vi "HEWH File Setup.vi"(0 "Data File Directory":path=path "D:/Data", 1 "Test_Type:":string(combo)="Stand Override", 2 "Station":string, 5 "error in (no error)":errorcluster, 7 "File Extension:":string="csv") -> (15 "FileInit Cluster":T8={"Scan Rate Adjust"=1000.0, "Draw Count"=0, "Test Patten Setup"={"Dispense Times"=[0.0, 3600.0, 7200.0, 10800.0, 14400.0, 18000.0], "Total Gallons Schedule"=[10.72, 10.72, 10.72, 10.72, 10.72, 10.72], "Flow Rate Schedule "=[3.0, 3.0, 3.0, 3.0, 3.0, 3.0], "Incoming Water Temperature"=[58.0, 58.0, 58.0, 58.0, 58.0, 58.0], "PreDraw Pattern"=[], "24 Hour PreDraw"=enum."Zero Pre-Draws", "Pre-Draw Until?"=[], "Purge Until Cutout"=FALSE, "Heating Flag"=FALSE}, "Condition Cluster Output"={"Condition #1"=FALSE, "Condition #2"=FALSE, "Special Last Draw (HU Test)"=FALSE, "RTD Out Temperature <="=0.0, "Condition #3"=FALSE, "Mean Tank Temperature <="=0.0, "Condition #4"=FALSE, "Decrease Outlet Temperature \nBy (RTD Out)"=0.0, "Condition #5"=FALSE, "Condition #6"=FALSE, "Time (Seconds)"=0.0, "Condition #7"=FALSE, "Condition #8"=FALSE, "Draw Until Condition"={"UE"=FALSE, "LE"=FALSE, "COMP"=FALSE, "FANS"=FALSE}, "Condition #9"=FALSE}, "HEWH Specific DAQ"={"HEWH Data"={"Voltage (Volts)"=-1.0, "Current (Amps)"=-1.0, "Power (Watts)"=-1.0, "WattHours (Wh)"=-1.0, "TC Tree (AVG)"=0.0, "Flow Rate (GPM)"=0.0, "Gallons (Gal)"=0.0, "RTD Out (Deg F)"=0.0, "TC Down"=0.0, "TC Tree Array"=[], "UE Event Lead"=0, "LE Event Lead"=0}, "Intellif Valve % Open"=0.0, "Power State"={"UE"=FALSE, "LE"=FALSE, "COMP"=FALSE, "FANS"=FALSE}, "Power Analyzer"=enum."APLUS", "Intellifaucet Configuration"=enum."DRK375,STATION3,1/2\"HOSE"}, "Test Output Data"={"PreDraw Data Table"=[], "Data Table"=[], "MW100 TC Headers"=[]}, "Calc and Calibration"={"RTD Max Min Array"=[], "Draw Statistics"=[], "Calibration Coefficients DBL"=[], "Min RTD Temp\nDuring Draw"=0.0, "Start Gallons"=0.0, "Starting Temp Decline Temp"=0.0, "Max RTD Temp\nDuring Draw"=0.0, "Draw Start Time"=0.0, "Delay Start Time"=0.0, "Current Purge Start Time"=0.0}, "Current Draw Time"=0.0} {"Test Patten Setup"."Incoming Water Temperature" format="%.2f"; "Test Patten Setup"."Flow Rate Schedule" format="%.2f"; "Test Patten Setup"."Total Gallons Schedule" format="%.2f"; "Test Patten Setup"."Dispense Times" format="%<%H:%M:%S>t"}, 19 "error out":errorcluster)   [LabVIEW 2016]
uses:
  Hybrid Water Heater/Type Definitions/HEWH Output Information.ctl
  Hybrid Water Heater/Type Definitions/HEWH Power Data.ctl
  Hybrid Water Heater/Type Definitions/HEWH Draw Pattern Setup.ctl
  Hybrid Water Heater/Type Definitions/HEWH Power Elements.ctl
  Hybrid Water Heater/Type Definitions/HEWH Termination Condition Cluster.ctl
  GEA2 Commands/HEWH/Type Definitions/GEA2 Commands.ctl
  Type Definitions/UTILITY Power Analyzer.ctl
  Hybrid Water Heater/Custom Instrument Control/Intellifaucet/Type Definitions/INTELLIFAUCET Tested Flowrate Scenarios.ctl
  File Setup.lvlib
  Type Definition/Save File DOE LabView Program.ctl
  LabVIEW GEA2 Toolkit v1.0.0.0/library/GEA2_Toolkit.lvlib
  Hybrid Water Heater/Type Definitions/HEWH Start Conditions.ctl
  Hybrid Water Heater/Support VIs/Draw Water Specific/Type Definitions/Terminate Draw Conditions.ctl
  Type Definition/Save File HEWH Heating Control Mode.ctl
  Hybrid Water Heater/Type Definitions/PRAT Test.ctl
  Hybrid Water Heater/Support VIs/Draw Water Specific/Type Definitions/HEWH Special Condition Check.ctl
  Hybrid Water Heater/Support VIs/Draw Water Specific/Type Definitions/Check Special Condtions.ctl
  Hybrid Water Heater/Type Definitions/HEWH Draw Flag ENUM.ctl
  Custom Pallet Controls/Custom Pallet String.ctl
  Custom Pallet Controls/Custom Pallet Forward.ctl
  Hybrid Water Heater/Type Definitions/HEWH PreDraw.ctl
  <vilib>/Platform/fileVersionInfo.llb/FileVersionInformation.ctl
  Type Definition/Save File DISH Dishwasher Details.ctl
  Type Definition/DPT IMC Data.ctl
  Washer DOE/Type Definitions/DOE Appliance Common.ctl
  Washer DOE/Type Definitions/DOE Dryer Standard.ctl
panel:
  in  "Appliance Details":T1={"FileVersionInfo"={"FileVersion"="", "ProductName"="", "InternalName"="", "CompanyName"="", "LegalCopyright"="", "FileDescription"=""}, "Dishwasher Info"={"Open Cup Weight (gm):"=0.0, "Auto Cup Weight (gm):"=0.0, "Detergent-Dish:"="", "Inlet Temperature-Dish:"="", "Cycle Mode-Dish:"="", "Unit Control-Dish:"="", "Manufacturer-Dish:"=""}, "Washer Info"={"Hot Water Temperature (Fahrenheit):"="", "Cold Water Temperature (Fahrenheit):"="", "Capacity (cu.ft):"=0.0, "Initial Cloth Weight:"=0.0, "Cloth Lot:"=0, "Model Family:"="", "Program Name:"="", "Cycle Selection:"="", "Wash Temperature:"="", "Rinse Temperature:"="", "Load Size:"=""}, "File Name Output Array"=[], "Calibration Output Array"=[], "Appliance Common"={"Engineer:"="", "Model Number:"="", "Serial Number:"="", "Comments:"="", "Station ID:"="", "Technician:"="", "TR Number:"="", "Lab ID:"="", "Voltage:"="", "Water Pressure (PSI):"="", "Test Date:"="", "Computer Name:"="", "IP Address:"="", "Ambient RH:"="", "Frequency:"="", "Build:"="", "Filename:"="", "Test Type:"="", "Load Run #:"=0, "Ambient Temperature (F):"="", "File Path:"=path "", "Cycles Per Year"=60}, "Water Heater"={"Heating Mode:"=""}, "Dryer"={"Heat Setting:"="", "Washer Water Temperature (60 ± 5°F):"=60, "Water Hardness (PPM):"=17, "Dryness Setting:"="", "Dryer Type:"="", "Exhaust:"="", "Drying Cycle:"="", "Load Type:"="", "Nominal Load Weight"="", "Dryer Initial IMC Data"={"Measured IMC (lbs)"=7.0, "Actual Initial RMC (%)"=7.0, "RMC (Desired %)"=100.0, "Bone Dry Wt(lbs)"=7.0, "Tolerance(%)"=5.0, "Actual Final RMC (%)"=7.0, "CEF (lbf/kWh)"=0.0, "Minimum Weight (lbf)"=0.0, "Average Weight (lbf)"=0.0, "Maximum Weight (lbf)"=0.0, "Measured IMC In Range?"=FALSE, "Moisture Reduction Factor"=55.5, "Field Use Factor"=1.04, "Empty Dryer Cold Weigth"=0.0, "Energy Standard"=enum."D2-Automatic Dryer", "Weight Cloth (lbs)"=0.0, "Relative Moisture Content (%)"=0.0, "Relative Moisture Content - Avg (%)"=0.0}}} {"Dryer"."Dryer Initial IMC Data"."Maximum Weight (lbf)" format="%03_6g"; "Dryer"."Dryer Initial IMC Data"."Average Weight (lbf)" format="%03_6g"; "Dryer"."Dryer Initial IMC Data"."Minimum Weight (lbf)" format="%03_6g"; "Dryer"."Dryer Initial IMC Data"."CEF (lbf/kWh)" format="%03_6g"; "Dryer"."Dryer Initial IMC Data"."Actual Final RMC (%)" format="%03_6g"; "Dryer"."Dryer Initial IMC Data"."Tolerance(%)" format="%0#_6g"; "Dryer"."Dryer Initial IMC Data"."Bone Dry Wt(lbs)" format="%03_6g"; "Dryer"."Dryer Initial IMC Data"."RMC (Desired %)" format="%0#_6g"; "Dryer"."Dryer Initial IMC Data"."Actual Initial RMC (%)" format="%03_6g"; "Dryer"."Dryer Initial IMC Data"."Measured IMC (lbs)" format="%0#_6g"}
  in  "Technician:":string(combo)
  in  "Lab ID:":string(combo)
  in  "TR Number:":string(combo)
  in  "Get Serial Number":bool
  in  "Get Model Number":bool
  in  "Supply Voltage":string(combo)
  in  "Heating Mode:":string(combo)
  out "Description":string="File Name Setup"
  in  "Model:":T4
  in  "Ambient Temp SetPoint:":string(combo)
  in  "Engineer:":T4
  in  "Comments:":string
  in  "Test Name:":T4
  in  "OK":T7
  in  "Serial Number:":T4
  in  "Ambient RH:":string(combo)
  in  "Build:":string(combo)
  in  "Frequency:":string(combo)
  in  "Test Station":T4
  in  "Tab Control":enum32{"Location Data", "Output Data"}(tab)
  out "Unhandled Error":errorcluster
  out "FileName":path
  out "Filename":string
  out "OutputData":string[][](array[string])
  # "Select Only One Condition"
  # "Just Draw Water!"
  # "Condition #1"
  # "Draw Until Any Heat Source"
  # "Condition #2"
  # "Start Dispense Pattern"
  # "Draw Until Specific Heat Source"
  # "Condition #3"
  # "Dispense PRAT Sequence"
  # "Not Working"
  # "Condition #4"
  # "Condition #5"
  # "Condition #6"
  # "Draw Pattern Setup"
  # "Pre-Draw Items"
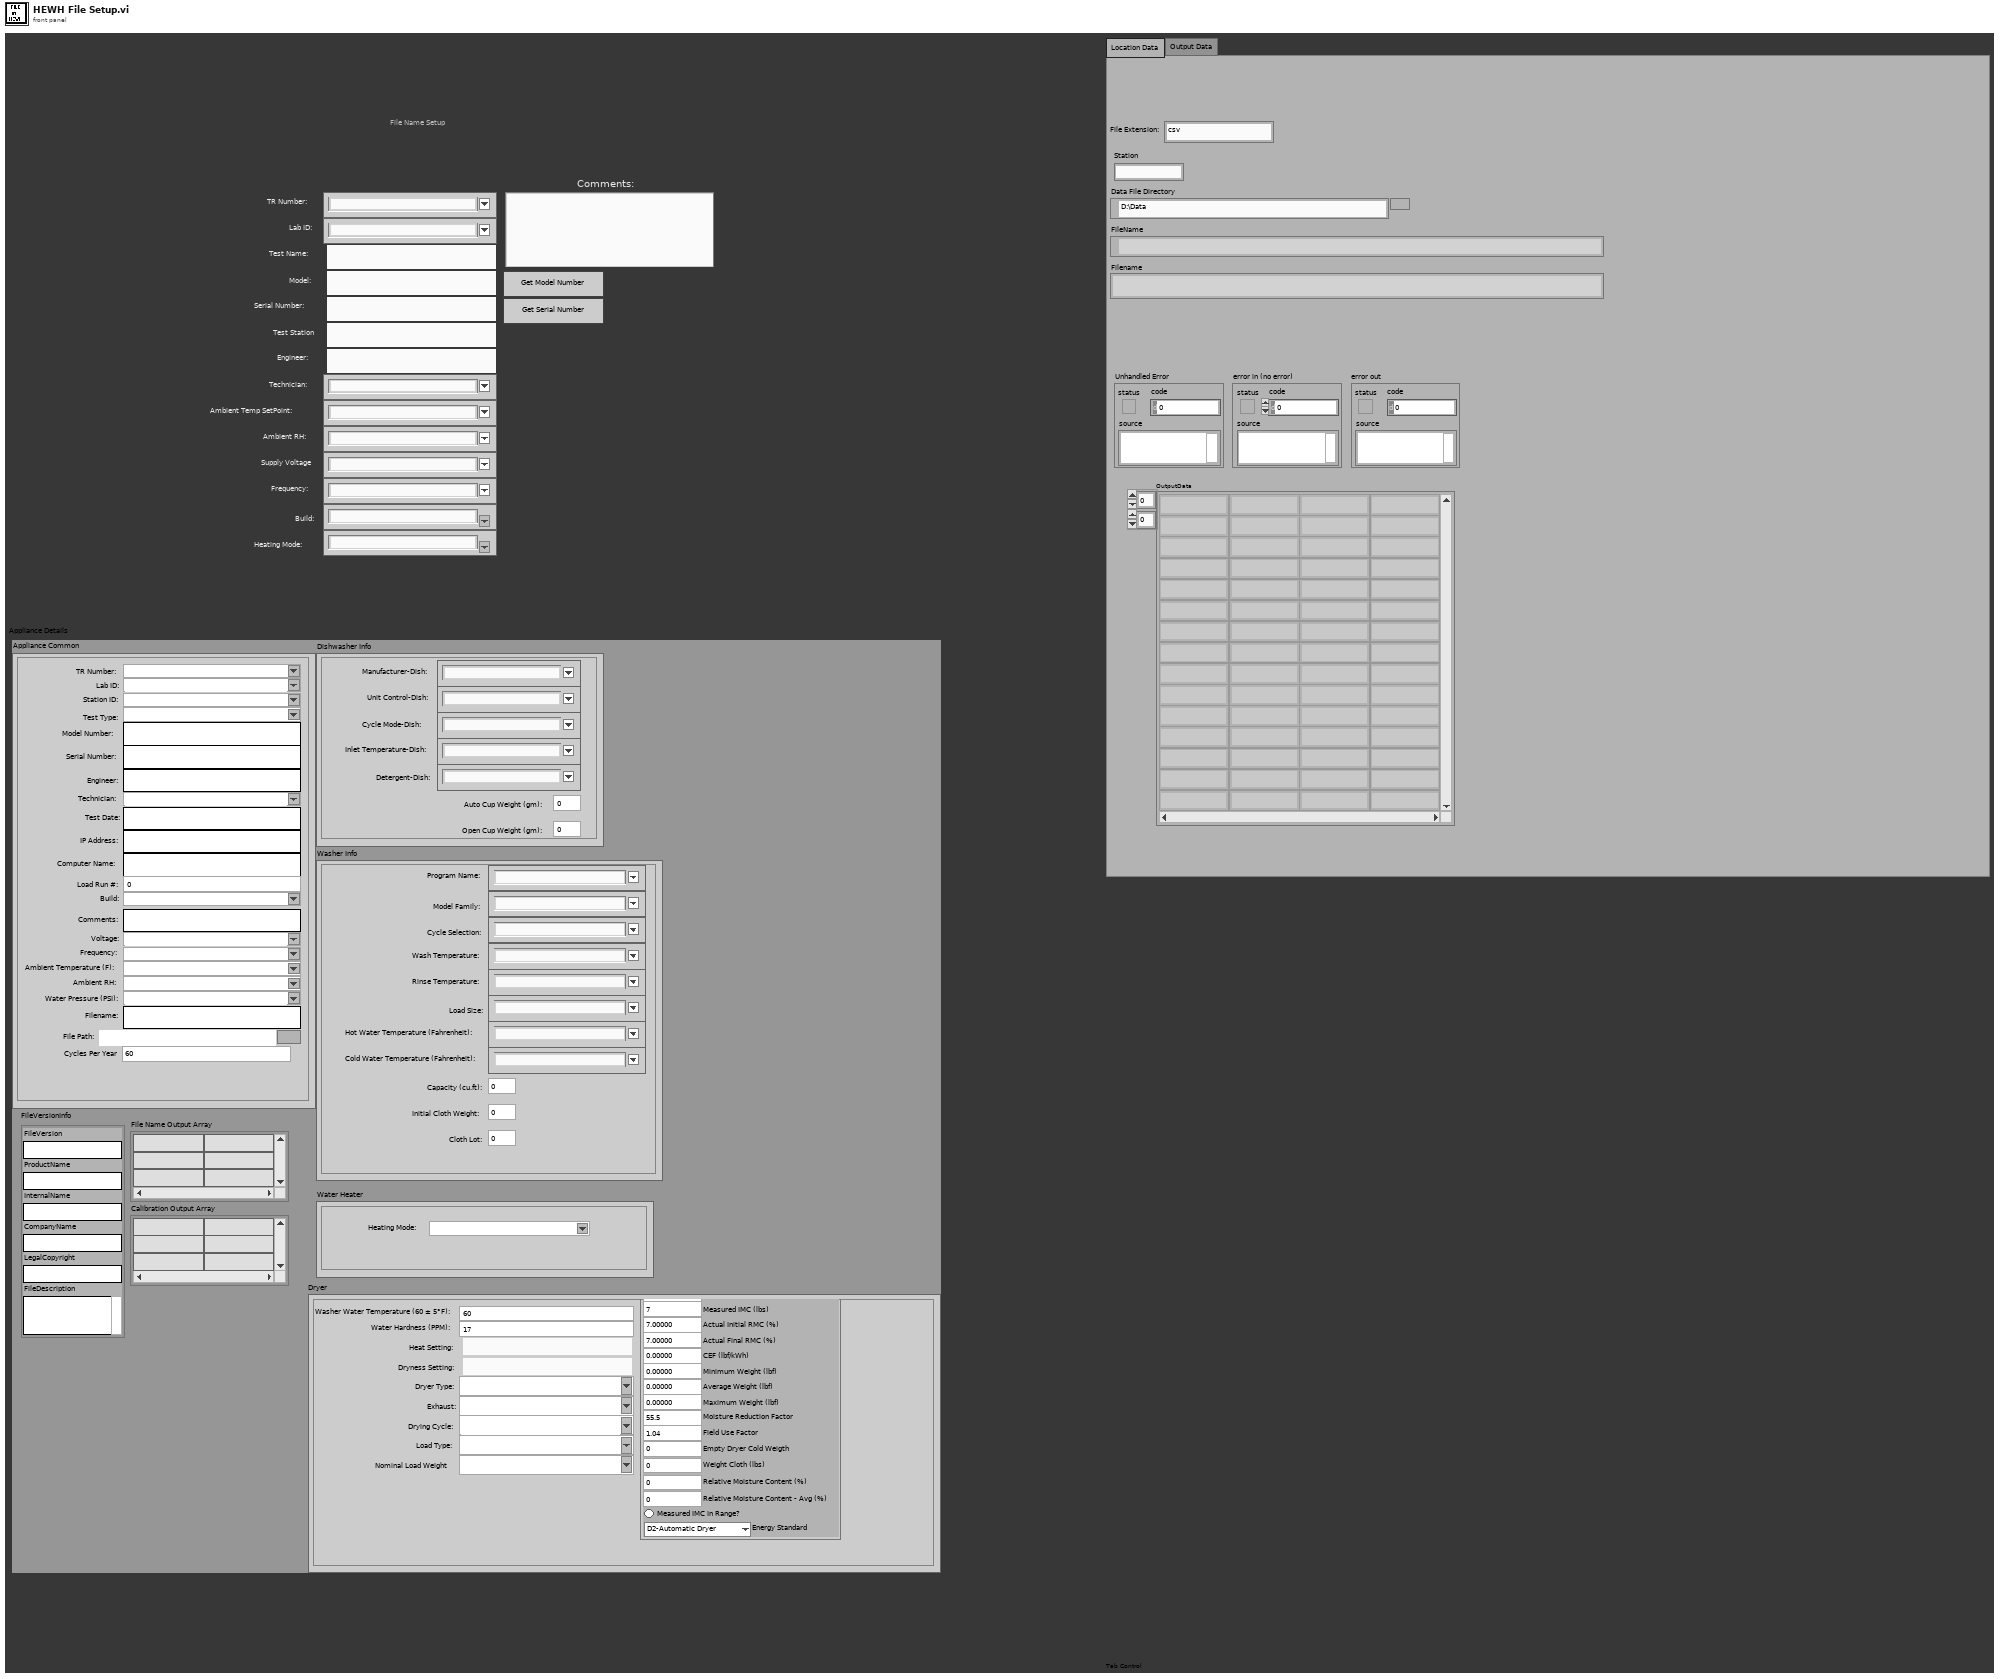
[diagram p1: front panel]
types:
  T1 = typedef "File Setup.lvlib/Save File DISH Dishwasher Details.ctl" = cluster{"FileVersionInfo":T2, "Dishwasher Info":cluster{"Open Cup Weight (gm):":dbl, "Auto Cup Weight (gm):":dbl, "Detergent-Dish:":string, "Inlet Temperature-Dish:":string, "Cycle Mode-Dish:":string, "Unit Control-Dish:":string, "Manufacturer-Dish:":string}, "Washer Info":cluster{"Hot Water Temperature (Fahrenheit):":string, "Cold Water Temperature (Fahrenheit):":string, "Capacity (cu.ft):":dbl, "Initial Cloth Weight:":dbl, "Cloth Lot:":i32, "Model Family:":string, "Program Name:":string, "Cycle Selection:":string, "Wash Temperature:":string, "Rinse Temperature:":string, "Load Size:":string}, "File Name Output Array":string[][], "Calibration Output Array":string[][], "Appliance Common":T3, "Water Heater":cluster{"Heating Mode:":string}, "Dryer":cluster{"Heat Setting:":T4, "Washer Water Temperature (60 ± 5°F):":u16, "Water Hardness (PPM):":u16, "Dryness Setting:":T4, "Dryer Type:":string, "Exhaust:":string, "Drying Cycle:":string, "Load Type:":string, "Nominal Load Weight":string, "Dryer Initial IMC Data":T5}}
  T2 = typedef "FileVersionInformation.ctl" = cluster{"FileVersion":string, "ProductName":string, "InternalName":string, "CompanyName":string, "LegalCopyright":string, "FileDescription":string}
  T3 = typedef "DOE Appliance Common.ctl" = cluster{"Engineer:":string, "Model Number:":string, "Serial Number:":string, "Comments:":string, "Station ID:":string, "Technician:":string, "TR Number:":string, "Lab ID:":string, "Voltage:":string, "Water Pressure (PSI):":string, "Test Date:":string, "Computer Name:":string, "IP Address:":string, "Ambient RH:":string, "Frequency:":string, "Build:":string, "Filename:":string, "Test Type:":string, "Load Run #:":i32, "Ambient Temperature (F):":string, "File Path:":path, "Cycles Per Year":u32}
  T4 = typedef "Custom Pallet String.ctl" = string
  T5 = typedef "DPT IMC Data.ctl" = cluster{"Measured IMC (lbs)":dbl, "Actual Initial RMC (%)":dbl, "RMC (Desired %)":dbl, "Bone Dry Wt(lbs)":dbl, "Tolerance(%)":dbl, "Actual Final RMC (%)":dbl, "CEF (lbf/kWh)":dbl, "Minimum Weight (lbf)":dbl, "Average Weight (lbf)":dbl, "Maximum Weight (lbf)":dbl, "Measured IMC In Range?":bool, "Moisture Reduction Factor":dbl, "Field Use Factor":dbl, "Empty Dryer Cold Weigth":dbl, "Energy Standard":T6, "Weight Cloth (lbs)":dbl, "Relative Moisture Content (%)":dbl, "Relative Moisture Content - Avg (%)":dbl}
  T6 = typedef "DOE Dryer Standard.ctl" = enum16{"D2-Automatic Dryer", "D2-Timer Dryer", "D1-Automatic Dryer", "D1-Timer Dryer", "Other"}
  T7 = typedef "Custom Pallet Forward.ctl" = bool
  T8 = typedef "HEWH Output Information.ctl" = cluster{"Scan Rate Adjust":dbl, "Draw Count":i32, "Test Patten Setup":T9, "Condition Cluster Output":T11, "HEWH Specific DAQ":cluster{"HEWH Data":T13, "Intellif Valve % Open":dbl, "Power State":T12, "Power Analyzer":T14, "Intellifaucet Configuration":T15}, "Test Output Data":cluster{"PreDraw Data Table":string[][], "Data Table":string[][], "MW100 TC Headers":string[]}, "Calc and Calibration":cluster{"RTD Max Min Array":dbl[][], "Draw Statistics":dbl[][], "Calibration Coefficients DBL":dbl[][], "Min RTD Temp\nDuring Draw":dbl, "Start Gallons":dbl, "Starting Temp Decline Temp":dbl, "Max RTD Temp\nDuring Draw":dbl, "Draw Start Time":dbl, "Delay Start Time":dbl, "Current Purge Start Time":dbl}, "Current Draw Time":dbl}
  T9 = typedef "HEWH Draw Pattern Setup.ctl" = cluster{"Dispense Times":dbl[], "Total Gallons Schedule":dbl[], "Flow Rate Schedule ":dbl[], "Incoming Water Temperature":dbl[], "PreDraw Pattern":dbl[][], "24 Hour PreDraw":T10, "Pre-Draw Until?":bool[], "Purge Until Cutout":bool, "Heating Flag":bool}
  T10 = typedef "HEWH PreDraw.ctl" = enum16{"Zero Pre-Draws", "One Pre- Draws", "Two Pre-Draws", "Three Pre-Draws", ""}
  T11 = typedef "HEWH Termination Condition Cluster.ctl" = cluster{"Condition #1":bool, "Condition #2":bool, "Special Last Draw (HU Test)":bool, "RTD Out Temperature <=":dbl, "Condition #3":bool, "Mean Tank Temperature <=":dbl, "Condition #4":bool, "Decrease Outlet Temperature \nBy (RTD Out)":dbl, "Condition #5":bool, "Condition #6":bool, "Time (Seconds)":dbl, "Condition #7":bool, "Condition #8":bool, "Draw Until Condition":T12, "Condition #9":bool}
  T12 = typedef "HEWH Power Elements.ctl" = cluster{"UE":bool, "LE":bool, "COMP":bool, "FANS":bool}
  T13 = typedef "HEWH Power Data.ctl" = cluster{"Voltage (Volts)":dbl, "Current (Amps)":dbl, "Power (Watts)":dbl, "WattHours (Wh)":dbl, "TC Tree (AVG)":dbl, "Flow Rate (GPM)":dbl, "Gallons (Gal)":dbl, "RTD Out (Deg F)":dbl, "TC Down":dbl, "TC Tree Array":dbl[], "UE Event Lead":i32, "LE Event Lead":i32}
  T14 = typedef "UTILITY Power Analyzer.ctl" = enum16{"", "APLUS", "WT210", "WT500", "WT300", "OSI", "Debug", "WT230", "WT300_1", "WT300_2"}
  T15 = typedef "INTELLIFAUCET Tested Flowrate Scenarios.ctl" = enum16{"DRK500,Station1", "DRK375,Lab", "SRK500,Station1,5GPM FR", "DRK375,STATION3,1/2\"HOSE", "DRK500,Station1,downspout", "DRK375,Station3,thruEcocute", "DRK375,Station3,purge", "Build2,2B,Purge", "Global, Purge", "Global, Tank", "DRK250"}
  T16 = enum32{"invalid app kind", "Development System", "Run Time System", "Student Edition", "Embedded LabVIEW", "Evaluation", "Custom"}
  T17 = enum32{"Invalid", "Standard", "Closed", "Hidden", "Minimized", "Maximized"}
  T18 = typedef "File Setup.lvlib/Save File DOE LabView Program.ctl" = enum16{"No Name Found", "DOE Stand", "Dishwasher Kitchen", "Portable Stand", "HEWH", "Dryer", "Dryer WILT", "HCC", "PRAT", "HEWH RLT"}
  T19 = typedef "GEA2 Commands.ctl" = enum16{"CMD_CANCEL_EEV_POSITION", "CMD_CLEAR_ENERGY_USAGE_CTRS", "CMD_CLEAR_FAULT_COUNTS", "CMD_CLEAR_OVERRIDE_STATUS", "CMD_COMP_OFF", "CMD_COMP_ON", "CMD_DSM_OVERRIDES", "CMD_EEV_POSITION", "CMD_ENTER_EXIT_FCT_MODE", "CMD_ENTER_FACT_MODE", "CMD_HP_RUN_6MIN", "CMD_INITIATE_REMOTE_DSM_OVERRIDE", "CMD_LE_2_SECONDS", "CMD_REFRESH_SERVICE_TIMEOUTS", "CMD_RESET", "CMD_RESET_FILTER_TIMES", "CMD_RESTORE_EEPROM_DEFAULTS", "CMD_RQST_LED_STATUS", "CMD_SET_AMBIENT_THRESH_1", "CMD_SET_AMBIENT_THRESH_2", "CMD_SET_AMBIENT_THRESH_3", "CMD_SET_CURRENTS", "CMD_SET_EEV_DRIVE_LINES", "CMD_SET_EEV_STOP_POSITION", "CMD_SET_LEDS", "CMD_SET_MODEL_NUMBER", "CMD_SET_PID_I_DENOM_OVER_THR", "CMD_SET_PID_I_DENOM_UNDER_THR", "CMD_SET_PID_LOW_SH_TARGET", "CMD_SET_PID_MID_SH_TARGET", "CMD_SET_PID_P_DENOMINATOR", "CMD_SET_SERIAL_NUMBER", "CMD_SET_START_POS_OVER_THR", "CMD_SET_START_POS_UNDER_THR", "CMD_TOGGLE_FAN", "CMD_TOGGLE_LE_SERV", "CMD_TOGGLE_SERVICE_MODE", "CMD_TOGGLE_UE_SERV", "CMD_TURN_ON_OFF_DLB", "CMD_UE_2_SECONDS", "CMD_UPDATE_DSM_LEVEL", "CMD_UPDATE_MODE", "CMD_WRITE_SETPOINTS", "REQ_READ_KEY_STATUS", "REQ_SYSTEM_MODE", "RQST_CURRENT_PID_SH_TARGET", "RQST_DATA_FROM_DATA_FLASH", "RQST_DATA_FROM_MEMORY", "RQST_DSM_OVERRIDE_STATUS", "RQST_HEM_KWH_DATA", "RQST_HYPERTERM_OUTPUT_DATA", "RQST_IDLB_RESISTANCE", "RQST_MODEL_NUMBER", "RQST_MODEL_SELECT_AD_VALUE", "RQST_OTHER_FAULT_COUNTS", "RQST_OVERRIDE_STATUS", "RQST_PID_PARAMETERS", "RQST_READ_PERSONALITY", "RQST_SERIAL_NUMBER", "RQST_SERVICE_ERROR_CODES", "RQST_Software_Version", "RQST_SS_FAULT_COUNTS", "RQST_STATUS_QUERY", "RQST_STD_ELEC_RANGE", "RQST_SUPPORTED_MODES", "RQST_T2_RESISTANCE", "RQST_T3B_RESISTANCE", "RQST_T4_RESISTANCE", "RQST_T5_RESISTANCE", "RQST_TEMP_RANGE", "RQST_VACATION_RANGE", "RQST_WATER_CAPACITY"}
  T20 = typedef "GEA2_Toolkit.lvlib/Data In.ctl" = cluster{"Source":u8, "Destination":u8, "Command":u8, "Message":string}
  T21 = typedef "GEA2_Toolkit.lvlib/Data Out.ctl" = cluster{"Source":u8, "Destination":u8, "Command":u8, "Length":u8, "CRC":u16, "Message":string}
  T22 = typedef "ViperHawk Data.ctl" = cluster{"GEA Diagnostic Data - Washer":T23, "Software Version":T24, "Debug Search Parameters":T25, "Message Count":i32, "Number of Messages":i32, "Partial Message String":string, "Full Message to Save":string, "Board ID":string, "Board Index":i32, "Source Address":u8, "Destination Address":u8, "Data to send":u8[], "ReceivedData":u8[], "Debug/GEA Data":string[], "Command":u8, "GEA2 Reference Out":refnum<k24>, "GEA2 Event Registration":refnum<event-registration>, "Bus Data":string, "GEA Data":string[][], "Network Variable Location":i32, "Water Heater GEA2 Data":T26}
  T23 = typedef "ViperHawk Diagnostic Data.ctl" = cluster{"Speed (RPM)":u32, "Load Size":u32, "Temperature":u32, "Water Pressure":dbl, "Detergent":u32, "Fabric Softener":u32, "Tub Direction":string, "Detergent Valve":bool, "Fabric Softener Valve":bool, "Recirculating Pump":bool, "Drain Valve":bool, "Hot Valve":bool, "Cold Valve":bool, "Lid Closed Status":string, "Lid Lock Status":string, "Error Count":u32, "IGBT Temperature (Deg C)":u32, "Motor Speed":u32, "Latched OOB":u32, "Raw OOB":u32, "Plaster Status":u32, "Inverter Power (W)":u32, "Target Speed(BRPM)":u32, "Latched Agitate Motor Temp (Deg C)":u32, "Current Motor Temp (Deg C)":u32, "Profiler Status":string, "Current Inverter Action":string, "Error Codes":string, "Lid Locked":bool, "Lid Closed":bool, "9E Diagnostic Data":cluster{"Total Cycle Time (Min)":u32, "Total Cycle Count (Current)":u16, "Total Error Count":u16, "Machine Error History":u32, "Washer UI History":u32, "Inverter Error History":u32, "Cycle Storage Limit":u8, "Error Storage Limit":u8, "Cycle Pages Supported":u8, "Error Pages Supported":u8, "Inverter Reset Count":u16}, "9F Diagnostic Data":cluster{"Cycle Buffer Index":string, "Page Number":string, "Total Cycle Count":u32, "Delay Start Time":u32, "Stain Selected":string, "Selected Cycle":u32, "eWash":string, "Soil Level":string, "Temperature":string, "Overnight Ready":string, "Spin Setting":string, "Control Lock Status":string, "Stain Remover":string, "Steam Assist":string, "My Cycle":string, "PreWash":string, "Debug Log Enabled":string, "Rinse":string, "Signal Level":string, "PreSoak":string}}
  T24 = typedef "Save File.lvlib/Save File Software Version.ctl" = cluster{"Critical Major SW Version":string, "Critical Minor SW Version":string, "Major SW Version":string, "Minor SW Version":string, "Parametric Data Ver. Major":string, "Parametric Data Ver. Minor":string, "Diagnostics Data Ver. Major":string, "Diagnostics Data Ver. Minor":string, "Current Personality Setting":string}
  T25 = typedef "ViperHawk Search Control.ctl" = cluster{"Pause":string[], "Run":string[], "EOC":string[], "Error Codes":string[]}
  T26 = typedef "GEA2 Commands WaterHeater GEA2 Data.ctl" = cluster{"GEA2 Label Array":string[], "PID_PARAMETERS":string[][], "SUPPORTED_MODES":string[][], "Button Status":T27, "Status Query":T28, "Service Error Codes":T29, "HEM_KWH_DATA":string[][], "OTHER_FAULT_COUNTS":string[][], "GEA2 Raw Message":string, "Hyperterminal Data":cluster{"Source":u8, "Destination":u8, "Command":u8, "Length":u8, "CRC":u16, "UE - state (1/0 on off)":u8, "LE - state (1/0 on off)":u8, "Comp - state (1/0 on off)":u8, "Fan  - state (1/0 on off)":u8, "Setpoint Deg F":i32, "T2(TankSensor)":dbl, "T3A(EvapIn)":dbl, "T3B(EvapOut)":dbl, "T4(CompressorDischarge)":dbl, "T5(Ambient)":dbl, "Current":dbl, "Voltage (Volts)":u16, "EEV Position (0-480)":u16, "Reason for last heating cycle termination":u16, "Reason Data word 1":string, "Reason Data word 2":string, "Reason Data word 3":string, "Reason Data word 4":string, "SW Debug Data":string, "Flow Events (Bit Encoded)":u16, "Heating Control Mode":u16}, "Extra Data":cluster{"Water Capacity (Gallons)":u32, "Max Vacation Duration Days":u32, "Min Vacation Duration Days":u32, "Max Set Point (Deg F)":u32, "Min Set Point (Deg F)":u32, "T5 Resistance":u32, "T4 Resistance":u32, "T3B Resistance":u32, "T2 Resistance":u32, "STD_ELEC_RANGE":string, "SS_FAULT_COUNTS":string, "SERIAL_NUMBER":string, "READ_PERSONALITY":u8, "RQST_OVERRIDE_STATUS":string, "MODEL_SELECT_AD_VALUE":u32, "MODEL NUMBER":string, "IDLB_RESISTANCE":u32, "DSM Override Status":string, "RQST_DATA_FROM_Memory":string, "RQST_DATA_FROM_DATA_FLASH":string, "RQST_CURRENT_PID_SH_TARGET":u16, "Unit System Mode":string}}
  T27 = typedef "GEA2 Commands Button Status.ctl" = cluster{"Switch 1":bool, "Switch 2":bool, "Switch 3":bool, "Switch 4":bool, "Switch 5":bool, "Switch 6":bool, "Switch 7":bool, "Switch 8":bool, "Switch 9":bool, "Switch 10":bool, "Switch 11":bool, "Switch 12":bool, "Switch 13":bool, "Switch 14":bool, "Switch 15":bool, "Switch 16":bool}
  T28 = typedef "GEA2 Commands Status Query.ctl" = cluster{"Days Remaining (For Std Electric and Vacation)":u8, "Unit Status":string, "Current Tank Temp in Deg F":u8, "Current Setpoint in Deg F":u8, "Filter Status (% used)":u8, "Fallback Status (Fallback heating mode)":string, "Fallback Temp":u8, "\"Set Mode\" Selection":string}
  T29 = typedef "GEA2 Commands Service Error Codes.ctl" = cluster{"Reserved":bool, "Reserved 1":bool, "Reserved 2":bool, "Reserved 3":bool, "Reserved 4":bool, "Reserved 5":bool, "Reserved 6":bool, "Reserved 7":bool, "DataFlash Fail Status":bool, "Stuck Key Fail Status":bool, "Dry Tank Fail Status":bool, "Miswire Fail Status":bool, "Reserved 8":bool, "Reserved 9":bool, "Reserved 10":bool, "Reserved 11":bool, "UE Fail Status":bool, "LE Fail Status":bool, "Filter Fail Status":bool, "T3A Fail Status":bool, "T3B Fail Status":bool, "T4 Fail Status":bool, "T5 Fail Status":bool, "T2 Fail Status":bool, "SS Cond A Status":bool, "SS Cond B Status":bool, "SS Cond C Status":bool, "SS Cond D Status":bool, "SS Cond E Status":bool, "SS Cond F Status":bool, "SS Fan Status":bool, "CMP Fail Status":bool}
  T30 = typedef "HEWH Output Information.ctl" = cluster{"Scan Rate Adjust":dbl, "Draw Count":i32, "Test Patten Setup":T31, "Condition Cluster Output":T11, "HEWH Specific DAQ":cluster{"HEWH Data":T39, "Intellif Valve % Open":dbl, "Power State":T12, "Power Analyzer":T14, "Intellifaucet Configuration":T15}, "Test Output Data":cluster{"PreDraw Data Table":string[][], "Data Table":string[][], "MW100 TC Headers":string[]}, "Calc and Calibration":cluster{"RTD Max Min Array":dbl[][], "Draw Statistics":dbl[][], "Calibration Coefficients DBL":dbl[][], "Min RTD Temp\nDuring Draw":dbl, "Start Gallons":dbl, "Starting Temp Decline Temp":dbl, "Max RTD Temp\nDuring Draw":dbl, "Draw Start Time":dbl, "Delay Start Time":dbl, "Current Purge Start Time":dbl}, "Current Draw Time":dbl}
  T31 = typedef "HEWH Draw Pattern Setup.ctl" = cluster{"Total Gallons Schedule":dbl[], "PRAT/RLT Sequence":T32[], "Current Sequence Index":i32}
  T32 = typedef "PRAT Test.ctl" = cluster{"Sequence #":dbl, "Cycles":i32, "Mode Setting":T33, "Flow Rate (GPM)":dbl, "Temperature (F)":dbl, "Reset Timer":bool, "Use Temp Decline Method":bool, "Terminate Condition":T34, "Condition Value #1":dbl, "UE":bool, "LE":bool, "Comp":bool, "Fan":bool, "Test End Time (Sec)":dbl, "Purge Until Cutout":bool, "Start Conditions":T35, "Condition Value #2":dbl, "Remove Power":bool, "Time":dbl, "Check Special Cond.":T36, "Condition#":T37, "Draw Flags":T38, "Data Processing Delay (FHD 15sec, UEF 5 Sec)":dbl, "Test Complete":bool}
  T33 = typedef "File Setup.lvlib/Save File HEWH Heating Control Mode.ctl" = string
  T34 = typedef "Terminate Draw Conditions.ctl" = enum16{"C1-Terminate Draw @ Gallon Mark", "C2-Special Last Draw (HU Test)", "C3-RTD Out <=", "C4-Mean Tank Temp <=", "C5-Decrease RTD Out (Deg F)", "C6-Time (Seconds)", "C7-Until Any Heat Source", "C8-Specific Heat Source", "C9-Do Nothing"}
  T35 = typedef "HEWH Start Conditions.ctl" = enum16{"Heat Source Cutout", "At Time (Seconds)", "Every X (Seconds)", "T2 >= X° Below Setpoint", "Seconds From Complete", "Wait for LE & Comp Cutout", "Wait for Comp Cutout", "Wait for LE Cutout", "Wait for UE Cutout"}
  T36 = typedef "Check Special Condtions.ctl" = enum16{"SC1-Do Nothing", "SC2-Check Heat Source (On-C2/Off-C1)", "SC3-Check Skip Condition", "SC4-Check Heat Source ON/Fail"}
  T37 = typedef "HEWH Special Condition Check.ctl" = enum16{"N/A", "C1", "C2", "Reset/Fail", "Skip Draw Sequence"}
  T38 = typedef "HEWH Draw Flag ENUM.ctl" = enum16{"N/A", "None(0)", "Sml(1)", "Med(2)", "SmlMed(3)", "Lrg(4)", "SmlLrg(5)", "MedLrg(6)", "SmlMedLrg(7)"}
  T39 = typedef "HEWH Power Data.ctl" = cluster{"HEWH Standard":cluster{"Voltage (Volts)":dbl, "Current (Amps)":dbl, "Power (Watts)":dbl, "WattHours (Wh)":dbl, "TC Tree (AVG)":dbl, "Flow Rate (GPM)":dbl, "Gallons (Gal)":dbl, "RTD Out (Deg F)":dbl, "RTD In (Deg F)":dbl, "RTD Amb (Deg F)":dbl, "TC Down":dbl, "UE Event Lead":i32, "LE Event Lead":i32, "TC Tree Array":dbl[]}, "PRAT":cluster{"Power (Watts) A":dbl, "Power (Watts) B":dbl, "Power (Watts) C":dbl, "Power (Watts) D":dbl, "TC1":dbl, "TC2":dbl, "TC3":dbl, "TC4":dbl, "WattHours (Wh) A":dbl, "WattHours (Wh) B":dbl, "WattHours (Wh) C":dbl, "WattHours (Wh) D":dbl, "Ambient":dbl, "Extra Temp":dbl}, "Additional Power Data":cluster{"Vthd":dbl, "Frequency (Hz)":dbl, "Apparent Power (VA)":dbl, "Power Factor":dbl, "Current Crest Factor":dbl, "Voltage Crest Factor":dbl, "Integration Time (sec)":dbl}}
  T40 = cluster{"Core":cluster{"Current VI Reference":refnum<vi>, "Close Panel on Exit?":bool}, "Error Flag":bool, "Weights":cluster{"Measured IMC":dbl, "Actual RMC":dbl, "RMC (Desired)":dbl, "Bone Dry Wt(lbs)":dbl, "Tolerance(%)":dbl}, "HEWH Output Information":T30, "Test_Type:":string, "Supply Voltage":string, "Appliance Details":T1}
  T41 = cluster{"Measured IMC":dbl, "Actual RMC":dbl, "RMC (Desired)":dbl, "Bone Dry Wt(lbs)":dbl, "Tolerance(%)":dbl}
  T42 = cluster{"Current VI Reference":refnum<vi>, "Close Panel on Exit?":bool}
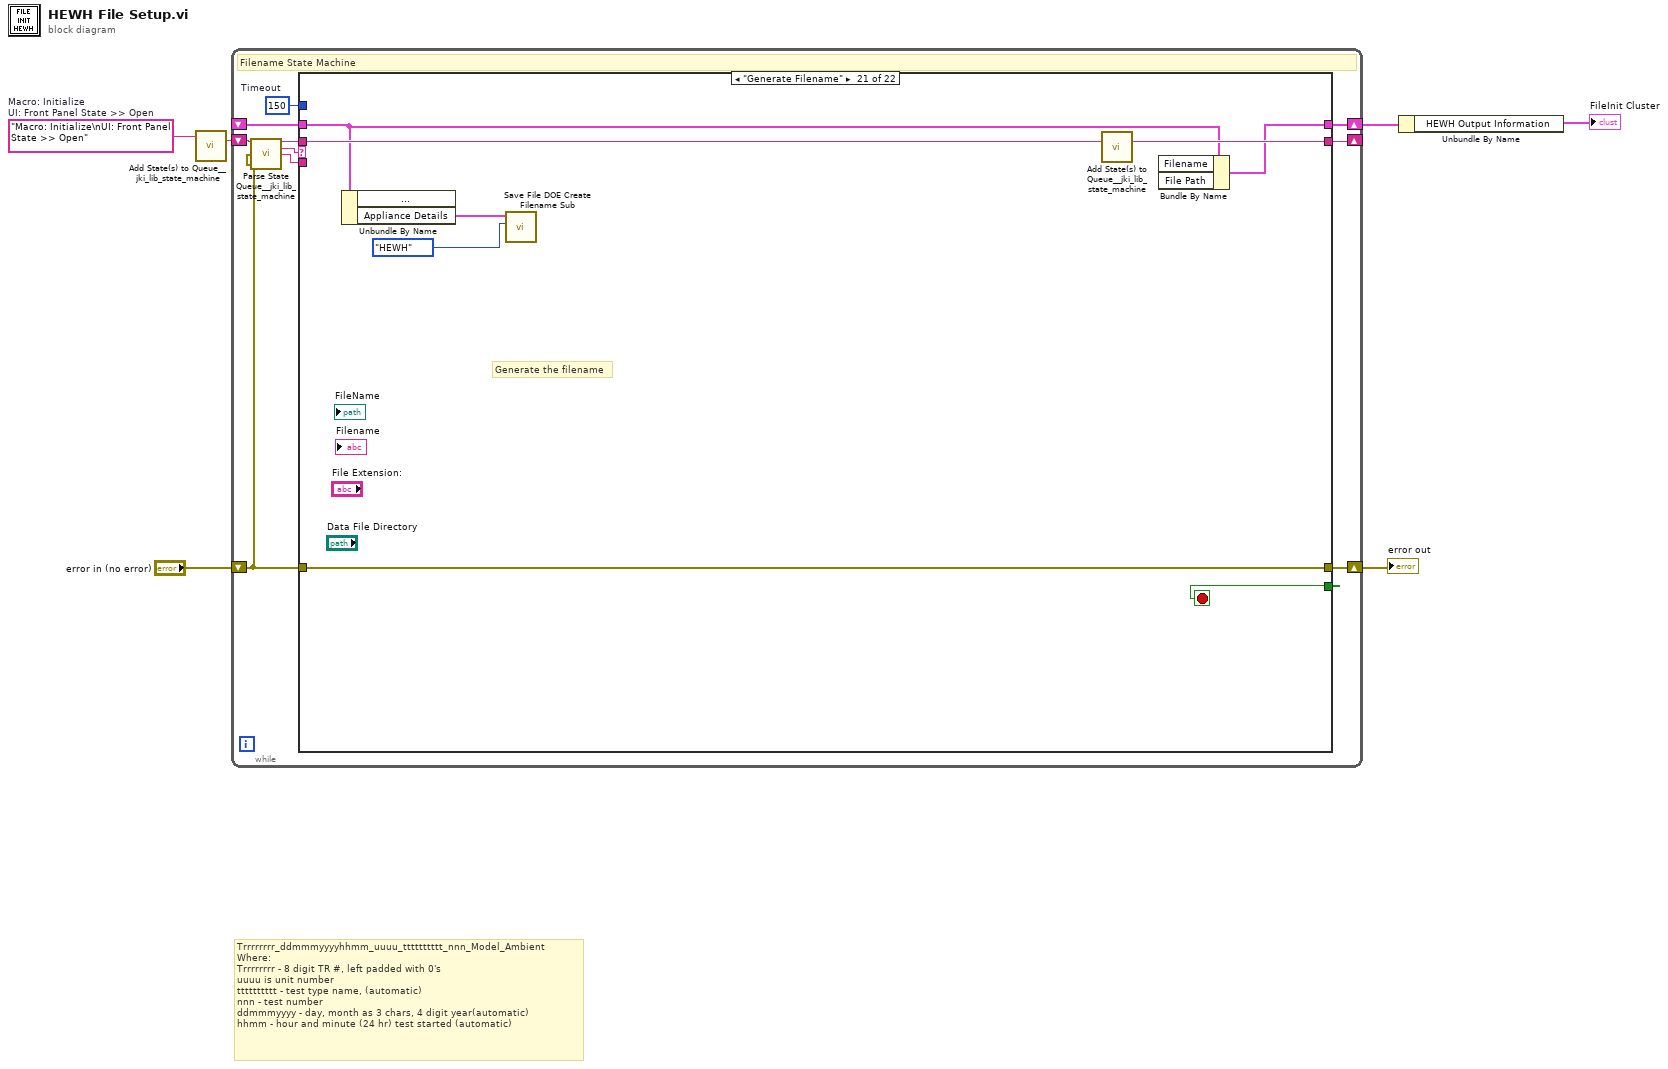
[diagram p0: block diagram]
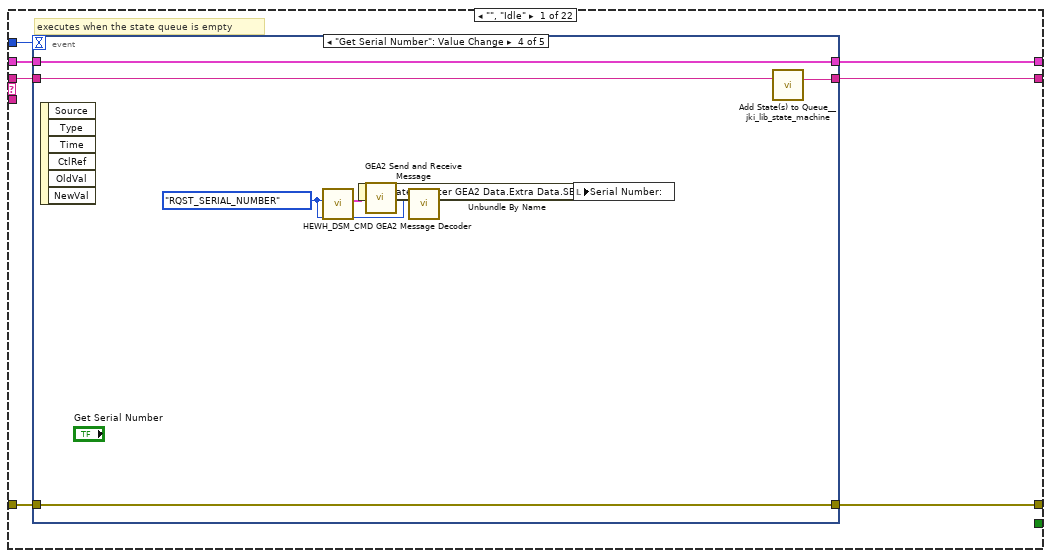
[diagram p2: hidden frame]
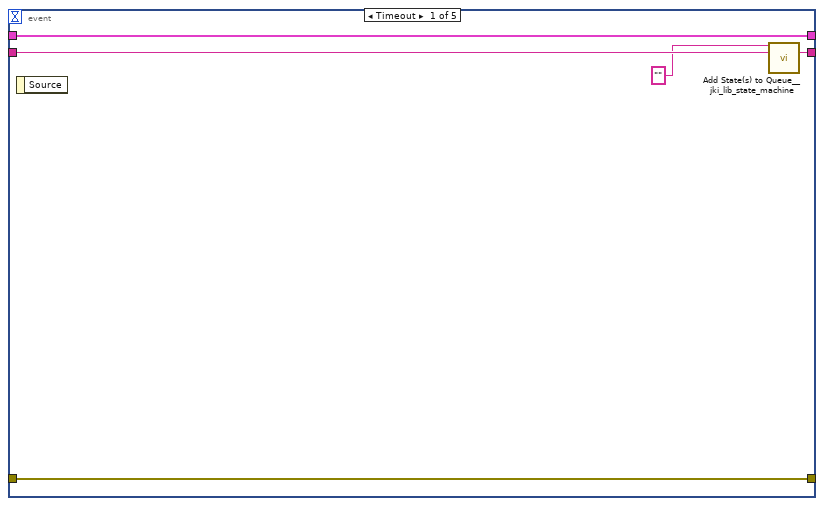
[diagram p3: hidden frame]
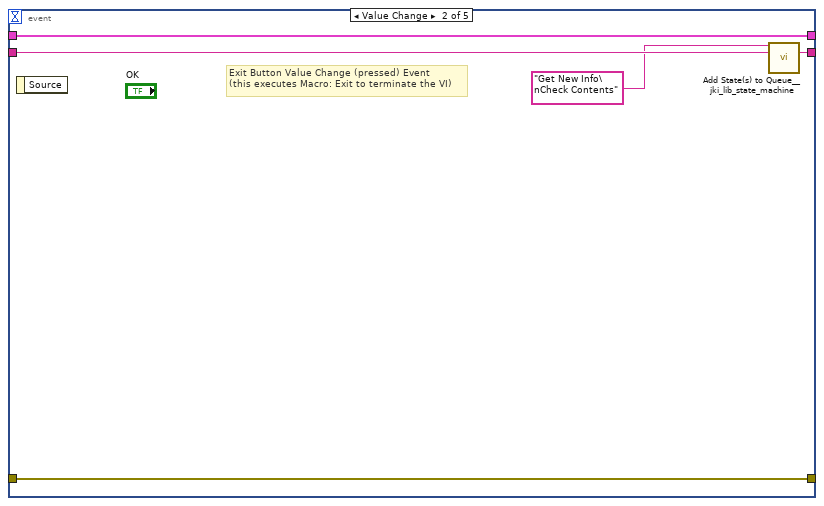
[diagram p4: hidden frame]
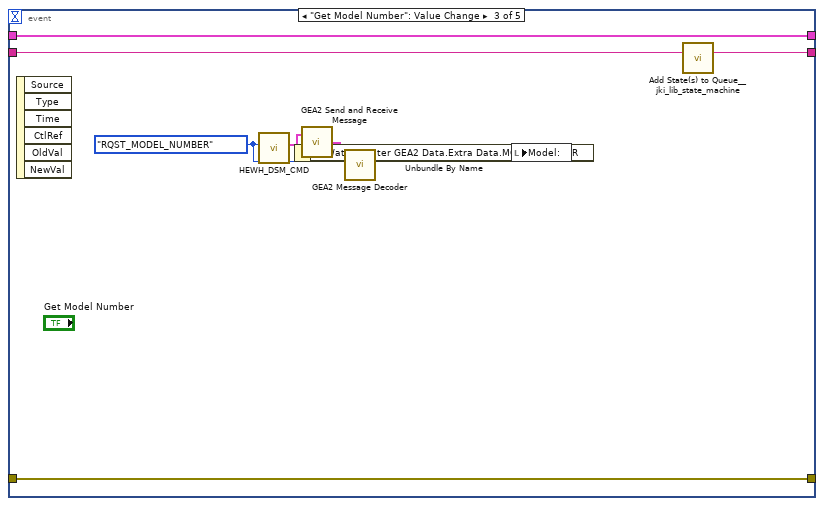
[diagram p5: hidden frame]
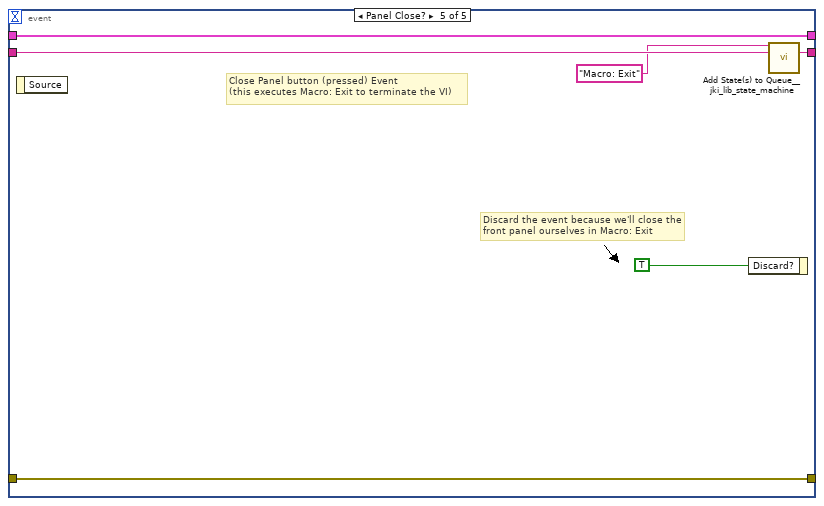
[diagram p6: hidden frame]
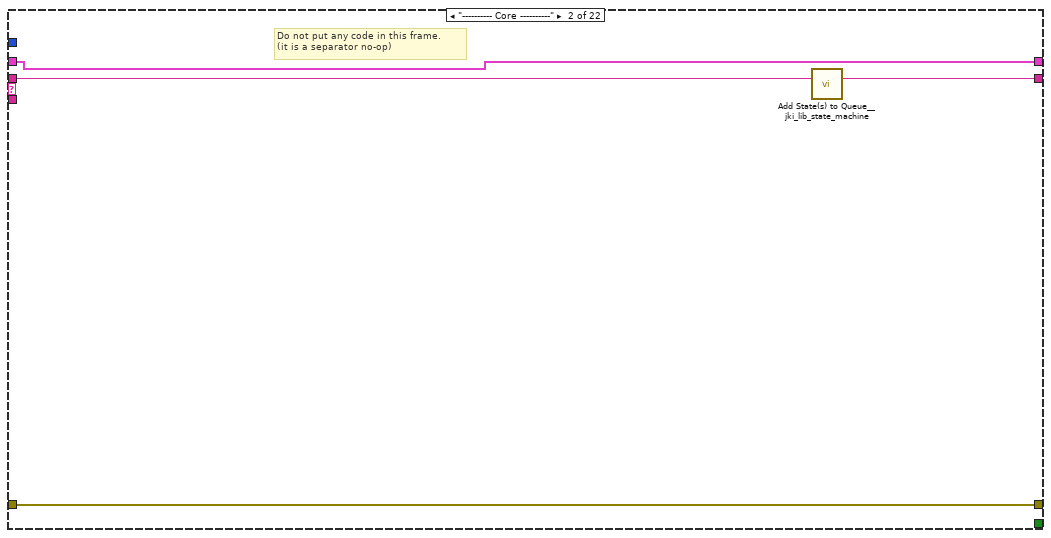
[diagram p7: hidden frame]
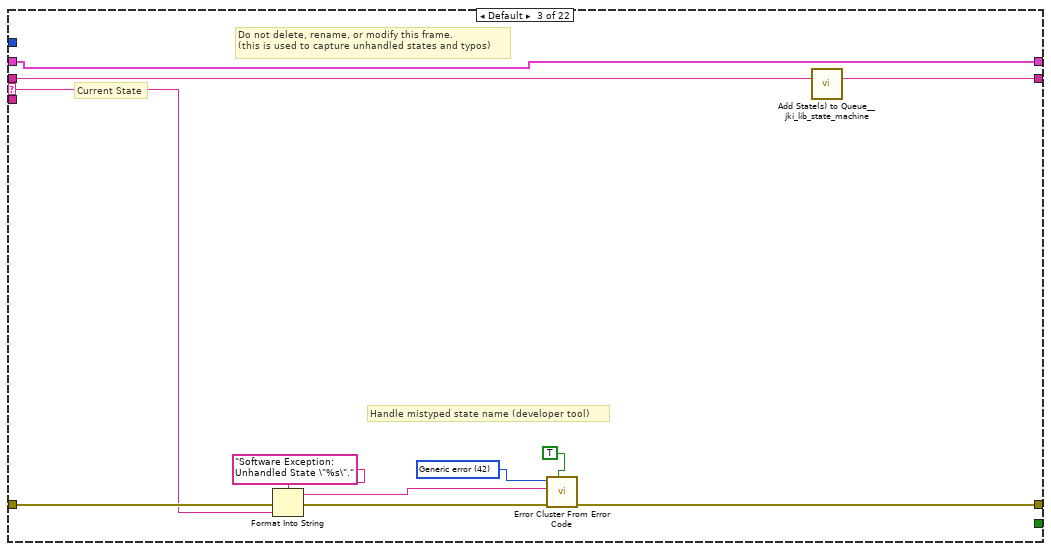
[diagram p8: hidden frame]
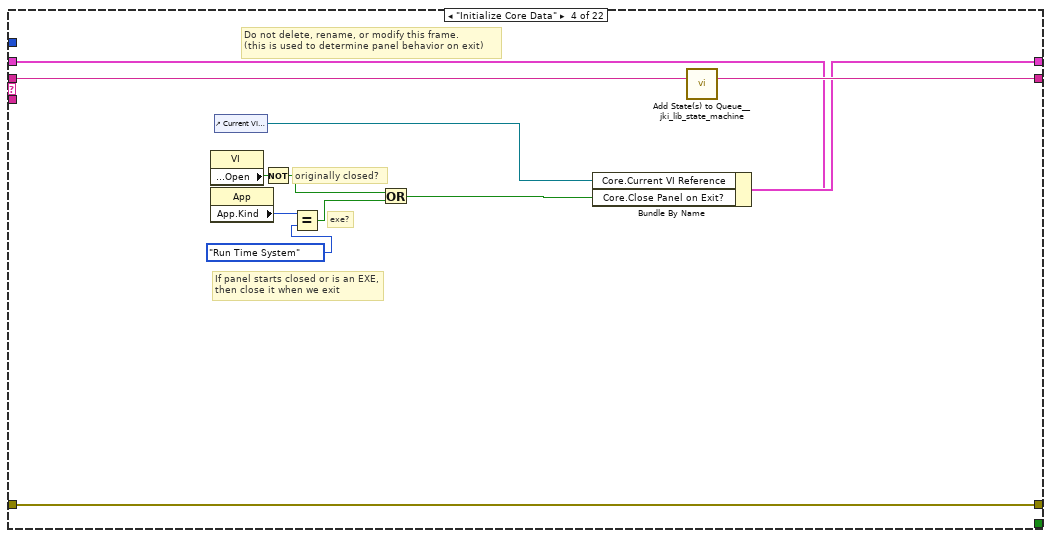
[diagram p9: hidden frame]
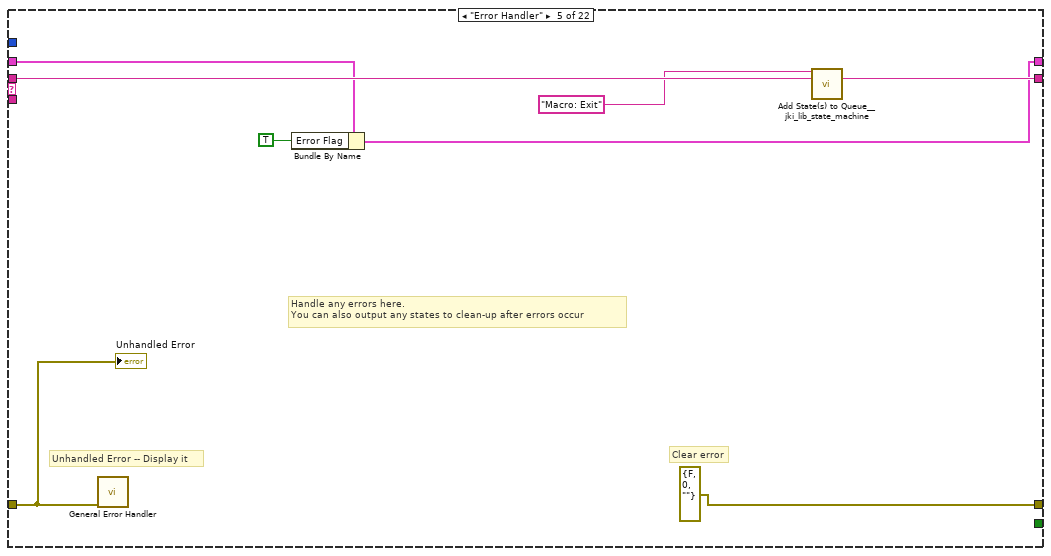
[diagram p10: hidden frame]
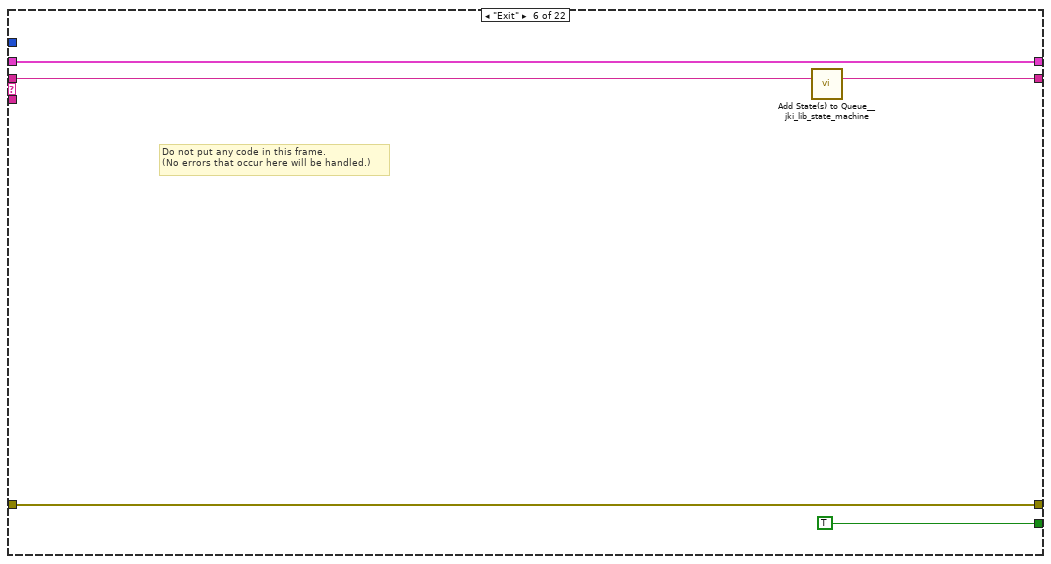
[diagram p11: hidden frame]
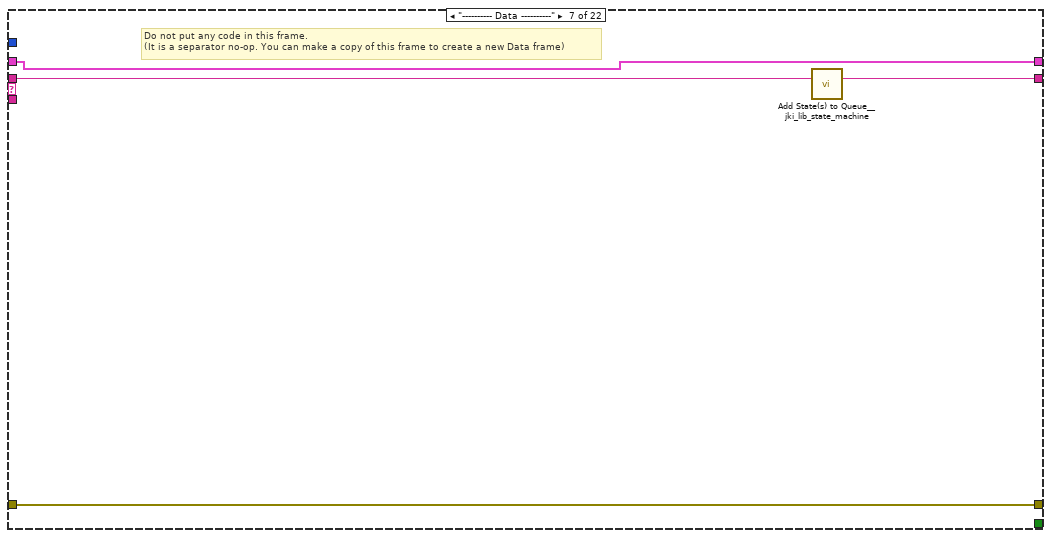
[diagram p12: hidden frame]
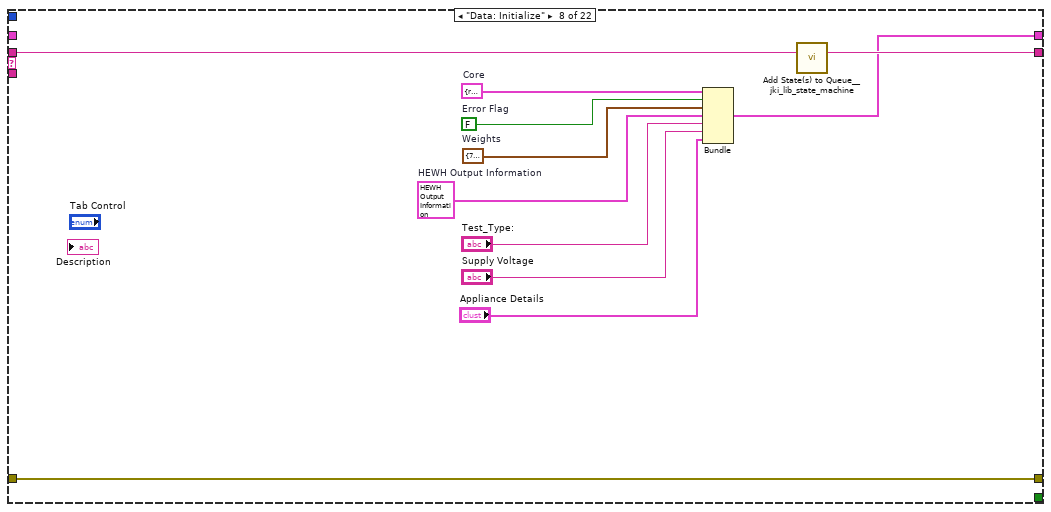
[diagram p13: hidden frame]
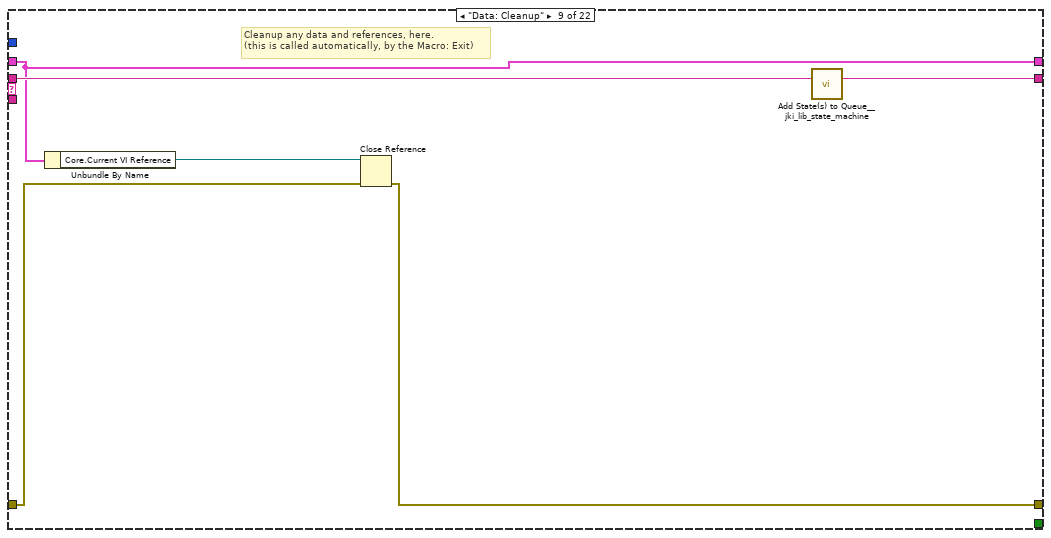
[diagram p14: hidden frame]
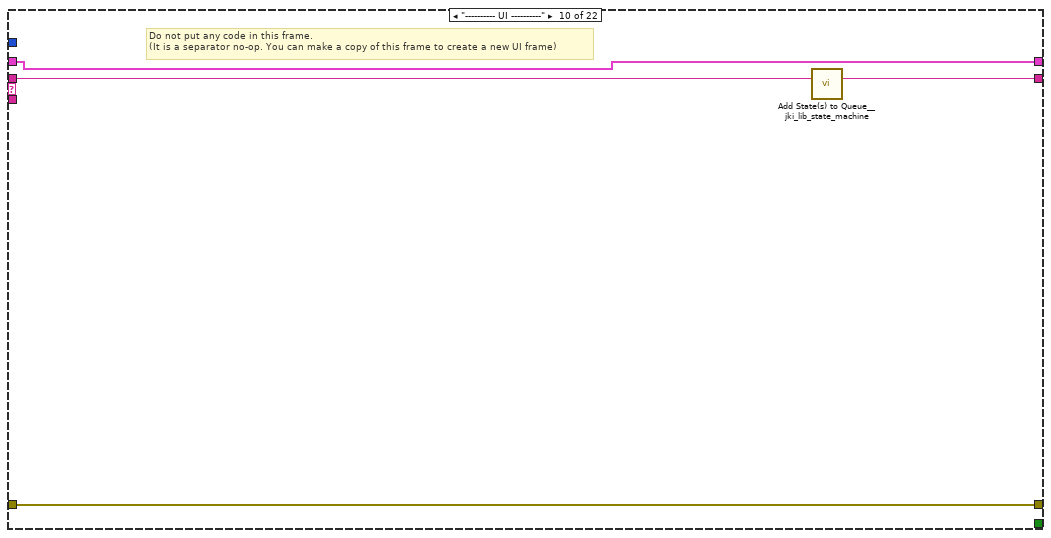
[diagram p15: hidden frame]
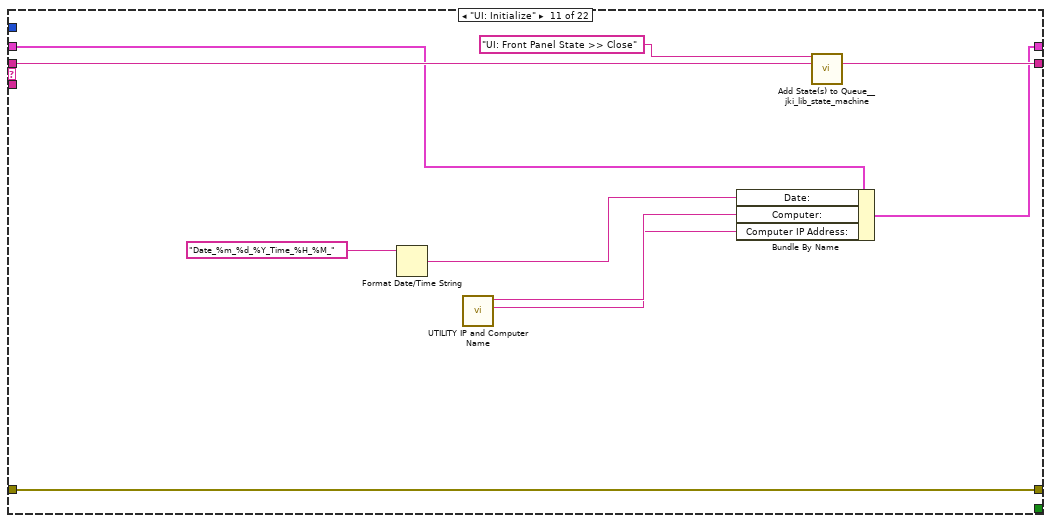
[diagram p16: hidden frame]
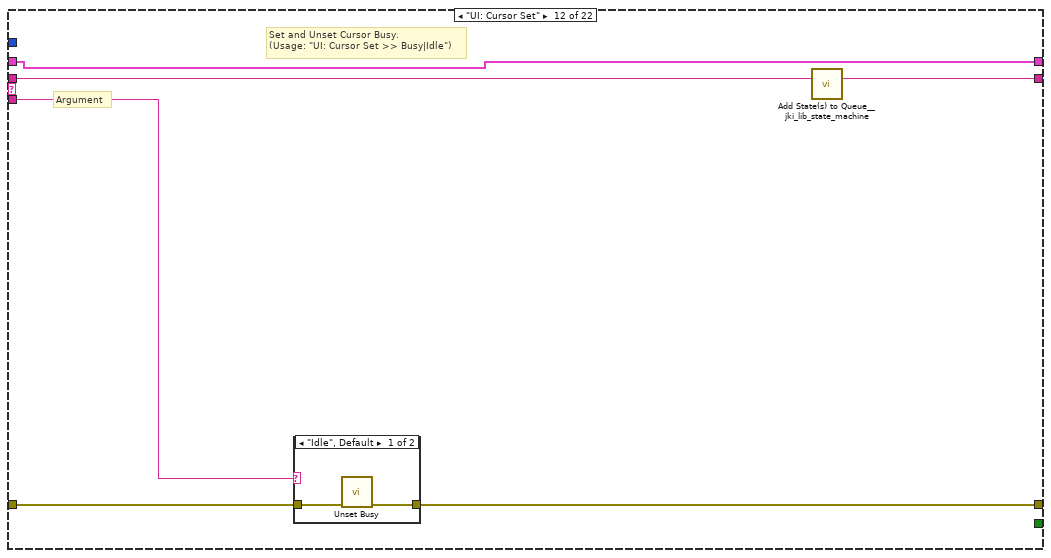
[diagram p17: hidden frame]
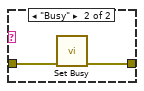
[diagram p18: hidden frame]
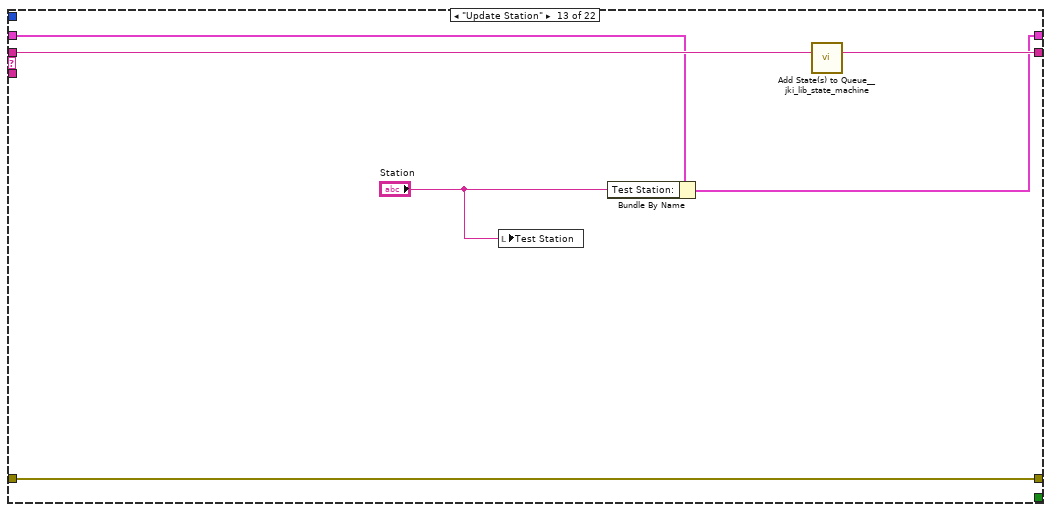
[diagram p19: hidden frame]
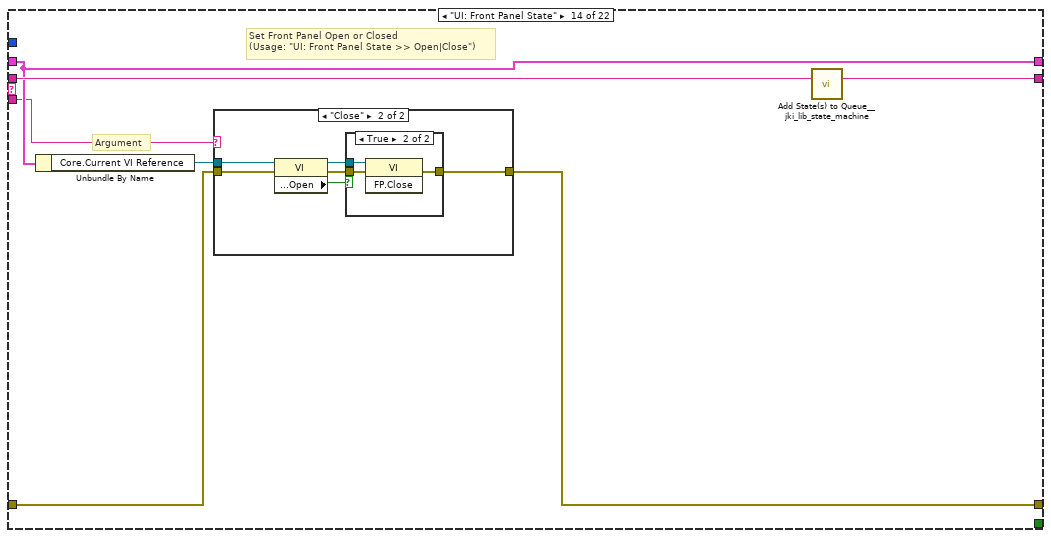
[diagram p20: hidden frame]
diagram:
  w4 = "Macro: Initialize\nUI: Front Panel State >> Open"  # Macro: Initialize UI: Front Panel State >> Open
  # "Trrrrrrrr_ddmmmyyyyhhmm_uuuu_tttttttttt_nnn_Model_Ambient\nWhere:\nTrrrrrrrr - 8 digit TR #, left padded with 0's\nuuuu is unit number\ntttttttttt - test type name, (automatic)\nnnn - test number\nddmmmyyyy - day, month as 3 chars, 4 digit year(automatic)\nhhmm - hour and minute (24 hr) test started (automatic)"
  n1 = call <vilib>:"Add State(s) to Queue__jki_lib_state_machine.vi"("State(s) in (\"\")"=w4) -> ("States Out"=w5:string)  [unwired: 14 in]
  n2 = while {
    shift-right: [w10] -> w1
    shift-left: _ -> [w9]
    shift-right: [w13] -> w6
    shift-left: "error in (no error)" -> [w7]
    shift-right: [w12] -> _
    shift-left: w5 -> [w14]
    stop <- w11 stop-if-true
    w8 = 150  # Timeout
    # "Filename State Machine"
    n3 = call <vilib>:"Parse State Queue__jki_lib_state_machine.vi"("State Queue"=w14, "Error In (no error)"=w7) -> ("Remaining States"=w16:string, "Current State"=w17:string, "Arguments"=w15:string)  [unwired: 11 in]
    n4 = case shown="\"Generate Filename\"" w17 {
      selector: w17 -> [_ _ w63 _ _ _ _ _ _ _ _ _ _ _ _ _ _ _ _ _ _ _]
      tunnel: w16 -> [w24 w62 w67 w85 w93 w98 w102 w113 w119 w123 w133 w139 w149 w156 w182 w189 w199 w203 w219 w246 w261 w274]
      tunnel: w15 -> [_ _ _ _ _ _ _ _ _ _ _ w134 _ w150 _ _ _ _ _ _ _ _]
      tunnel: w9 -> [w22 w59 w65 w76 w88 w96 w99 _ w114 w120 w129 w137 w146 w152 w179 w186 w196 w200 w221 w242 w259 w268]
      tunnel: [w21 w60 w69 w82 errorcluster {"status"=FALSE, "code"=0, "source"=""} ("error out") w95 w100 w110 w115 w121 w131 w135 w147 w153 w180 w187 w197 w201 w222 w244 w255 w271] -> w13
      tunnel: w7 -> [w20 w60 w68 w82 w90 w95 w100 w110 w116 w121 w131 w136 w147 w154 w180 w187 w197 w201 w222 w244 w255 w272]
      tunnel: [w23 w61 w66 w84 w92 w97 w101 w112 w118 w122 w132 w138 w148 w155 w181 w188 w198 w202 w223 w245 w260 w273] -> w12
      tunnel: [_ _ _ _ _ TRUE _ _ _ _ _ _ _ _ _ _ _ _ _ _ _ _] -> w11
      tunnel: [w19 w59 w65 w83 w87 w96 w99 w111 w114 w120 w128 w137 w145 w152 w179 w186 w196 w200 w220 w241 w258 w267] -> w10
      tunnel: w8 -> [w18 _ _ _ _ _ _ _ _ _ _ _ _ _ _ _ _ _ _ _ _ _]
      frame "", "Idle" {
        # "executes when the state queue is empty"
        n5 = event shown="[3] \"Get Serial Number\": Value Change" {
          selector: _ -> [_ _ _ _ _]
          dyn-events: _ -> [_ _ _ _ _]
          timeout: w18 -> [_ _ _ _ _]
          tunnel: w24 -> [w29 w34 w40 w46 w58]
          tunnel: [w28 w33 w41 w47 w57] -> w23
          tunnel: w22 -> [w26 w31 w42 w48 w55]
          tunnel: [w27 w32 w43 w49 w56] -> w21
          tunnel: w20 -> [w27 w32 w43 w49 w56]
          tunnel: [w26 w31 w42 w48 w55] -> w19
          event Timeout {
            n6 = event-data() -> ()  [unwired: 1 in, 1 out]
            n7 = call <vilib>:"Add State(s) to Queue__jki_lib_state_machine.vi"("State(s) in Front (\"\")"="" ("State(s) in Front (\"\")"), "State(s) in (\"\")"=w29) -> ("States Out"=w28:string)  [unwired: 13 in]
          }
          event Value Change {
            # "Exit Button Value Change (pressed) Event\n(this executes Macro: Exit to terminate the VI)"
            n8 = event-data() -> ()  [unwired: 1 in, 1 out]
            n9 = call <vilib>:"Add State(s) to Queue__jki_lib_state_machine.vi"("State(s) in Front (\"\")"="Get New Info\nCheck Contents", "State(s) in (\"\")"=w34) -> ("States Out"=w33:string)  [unwired: 13 in]
          }
          event "Get Model Number": Value Change {
            w39 = GEA2_Commands."RQST_MODEL_NUMBER" ("GEA2 Commands and Requests")
            n10 = event-data() -> ()  [unwired: 1 in, 6 out]
            n11 = call "HEWH_DSM_CMD.vi"("GEA2 Commands and Requests"=w39) -> ("Input Data"=w36:T20)  [unwired: 8 in, 1 out]
            n12 = call "GEA2 Send and Receive Message.vi"("Input Data"=w36) -> ("Converted Data Out"=w35:T21)  [unwired: 9 in, 5 out]
            n13 = call "GEA2 Message Decoder.vi"("GEA2 Commands and Requests"=w39, "Coverted Data Out"=w35) -> ("GEA Information Out"=w38:T22)  [unwired: 9 in]
            n14 = Unbundle By Name(w38) -> ("Water Heater GEA2 Data.Extra Data.MODEL NUMBER"=w37:string)
            n15 = local write "Model:"(w37) -> ()
            n16 = call <vilib>:"Add State(s) to Queue__jki_lib_state_machine.vi"("State(s) in (\"\")"=w40) -> ("States Out"=w41:string)  [unwired: 14 in]
          }
          event "Get Serial Number": Value Change {
            w52 = GEA2_Commands."RQST_SERIAL_NUMBER" ("GEA2 Commands and Requests")
            n17 = event-data() -> ()  [unwired: 1 in, 6 out]
            n18 = call "HEWH_DSM_CMD.vi"("GEA2 Commands and Requests"=w52) -> ("Input Data"=w45:T20)  [unwired: 8 in, 1 out]
            n19 = call "GEA2 Send and Receive Message.vi"("Input Data"=w45) -> ("Converted Data Out"=w44:T21)  [unwired: 9 in, 5 out]
            n20 = call "GEA2 Message Decoder.vi"("GEA2 Commands and Requests"=w52, "Coverted Data Out"=w44) -> ("GEA Information Out"=w51:T22)  [unwired: 9 in]
            n21 = Unbundle By Name(w51) -> ("Water Heater GEA2 Data.Extra Data.SERIAL_NUMBER"=w50:string)
            n22 = local write "Serial Number:"(w50) -> ()
            n23 = call <vilib>:"Add State(s) to Queue__jki_lib_state_machine.vi"("State(s) in (\"\")"=w46) -> ("States Out"=w47:string)  [unwired: 14 in]
          }
          event Panel Close? {
            # "Discard the event because we'll close the front panel ourselves in Macro: Exit"
            # "Close Panel button (pressed) Event\n(this executes Macro: Exit to terminate the VI)"
            n24 = event-data() -> ()  [unwired: 1 in, 1 out]
            n25 = event-data("Discard?"=TRUE) -> ()  [unwired: 1 in, 1 out]
            n26 = call <vilib>:"Add State(s) to Queue__jki_lib_state_machine.vi"("State(s) in Front (\"\")"="Macro: Exit", "State(s) in (\"\")"=w58) -> ("States Out"=w57:string)  [unwired: 13 in]
          }
        }
      }
      frame "---------- Core ----------" {
        # "Do not put any code in this frame.\n(it is a separator no-op)"
        n27 = call <vilib>:"Add State(s) to Queue__jki_lib_state_machine.vi"("State(s) in (\"\")"=w62) -> ("States Out"=w61:string)  [unwired: 14 in]
      }
      frame Default {
        w72 = 42 items=["No error", "Argument error", "Memory is full", "Out of zone", "End of file", "File already open", "Generic file I/O error", "File not found", "File permission error", "Disk is full", "Duplicate path", "Too many files open", "System feature not enabled", "Resource file not found", "Cannot add resource", "Resource not found", "Image not found", "Image memory error", "Pen does not exist", "Config type invalid", "Config token not found", "Config parse error", "Config memory error", "Bad external code format", "Bad external code offset", "External code not present", "Null window", "Destroy window error", "Null menu", "Print aborted", "Bad print record", "Print driver error", "Windows error during printing", "Memory error during printing", "Print dialog error", "Generic print error", "Invalid device refnum", "Device not found", "Device parameter error", "Device unit error", "Cannot open device", "Device call aborted", "Generic error", "Cancelled by user", "Object ID too low", "Object ID too high", "Object not in heap", "Unknown heap", "Unknown object (invalid DefProc)", "Unknown object (DefProc not in table)", "Message out of range", "Invalid (null) method", "Unknown message", "Manager call not supported", "Bad address", "Network operation in progress", "Network operation timed out", "Connection is busy", "Network attribute not supported", "Network error", "Address in use", "System out of memory", "Connection aborted", "Connection refused", "Not connected", "Already connected", "Connection closed", "Initialization error (interapplication manager)", "Bad occurrence", "Wait on unbound occurrence handler", "Occurrence queue overflow", "Datalog type conflict", "Unused", "Unrecognized type (interapplication manager)", "Memory corrupt", "Failed to make temporary DLL", "Old CIN version", "Drag socket not found", "Failed to load drop-object", "Failed to register OLE object", "Failed to release OLE object", "Format specifier type mismatch", "Unknown format specifier", "Too few format specifiers", "Too many format specifiers", "Scan failed", "Newer CIN version", "Error converting to variant", "Runtime menu error", "Password tampered", "Variant attribute not found", "Incompatible variant data type", "Event data is not available", "Event Store is not present", "Occurrence is not found", "Event Queue is not created", "Event info is not available", "Refnum passed is NULL", "Error retrieving Class GUID", "Error retrieving CoClass GUID", "Error retrieving TypeLib GUID.", "Bad built application magic bytes.", "Specific driver is different from the specific driver associated with the Logical Name.", "There is no session opened to the class driver.", "Max Error", "MAX - Error with config objects", "MAX - Error loading configuration", "MAX - Group not supported"]
        # "Current State"
        # "Do not delete, rename, or modify this frame.\n(this is used to capture unhandled states and typos)"
        # "Handle mistyped state name (developer tool)"
        n28 = Format Into String(format string="Software Exception: Unhandled State \"%s\"." ("message"), error in=w68, w63) -> (resulting string=w71:string, error out=w70:errorcluster)  [unwired: 1 in]
        n29 = call <vilib>:"Error Cluster From Error Code.vi"("show call chain? (False)"=TRUE, "error in (no error)"=w70, "error message (\"\")"=w71, "error code (0)"=w72) -> ("error out"=w69:errorcluster)  [unwired: 5 in]
        n30 = call <vilib>:"Add State(s) to Queue__jki_lib_state_machine.vi"("State(s) in (\"\")"=w67) -> ("States Out"=w66:string)  [unwired: 14 in]
      }
      frame "Initialize Core Data" {
        # "Do not delete, rename, or modify this frame.\n(this is used to determine panel behavior on exit)"
        # "originally closed?"
        # "exe?"
        # "If panel starts closed or is an EXE, then close it when we exit"
        n31 = property class="VI"() -> ("Front Panel.Open"=w81:bool)  [unwired: 2 in, 2 out]
        n32 = property class="App"() -> ("App.Kind"=w80:T16)  [unwired: 2 in, 2 out]
        n33 = control-ref of="Current VI Reference"() -> (w74:refnum<vi>)
        n34 = Not(x=w81) -> (.not. x?=w78:bool)
        n35 = Equal?(x=w80, y=T16."Run Time System" ("Application:Kind")) -> (x = y?=w77:bool)
        n36 = Or(x=w78, y=w77) -> (x .or. y?=w75:bool)
        n37 = Bundle By Name(cluster=w76, "Core.Current VI Reference"=w74, "Core.Close Panel on Exit?"=w75) -> (w83:T40)
        n38 = call <vilib>:"Add State(s) to Queue__jki_lib_state_machine.vi"("State(s) in (\"\")"=w85) -> ("States Out"=w84:string)  [unwired: 14 in]
      }
      frame "Error Handler" {
        # "Unhandled Error -- Display it"
        # "Handle any errors here.\nYou can also output any states to clean-up after errors occur"
        # "Clear error"
        n39 = call <vilib>:"General Error Handler.vi"("error in (no error)"=w90) -> ()  [unwired: 10 in, 5 out]
        n40 = Bundle By Name(cluster=w88, "Error Flag"=TRUE) -> (w87:T40)
        n41 = call <vilib>:"Add State(s) to Queue__jki_lib_state_machine.vi"("State(s) in Front (\"\")"="Macro: Exit", "State(s) in (\"\")"=w93) -> ("States Out"=w92:string)  [unwired: 13 in]
        "Unhandled Error" <- w90
      }
      frame "Exit" {
        # "Do not put any code in this frame.\n(No errors that occur here will be handled.)"
        n42 = call <vilib>:"Add State(s) to Queue__jki_lib_state_machine.vi"("State(s) in (\"\")"=w98) -> ("States Out"=w97:string)  [unwired: 14 in]
      }
      frame "---------- Data ----------" {
        # "Do not put any code in this frame.\n(It is a separator no-op. You can make a copy of this frame to create a new Data frame)"
        n43 = call <vilib>:"Add State(s) to Queue__jki_lib_state_machine.vi"("State(s) in (\"\")"=w102) -> ("States Out"=w101:string)  [unwired: 14 in]
      }
      frame "Data: Initialize" {
        w106 = T30 {"Scan Rate Adjust"=0.0, "Draw Count"=0, "Test Patten Setup"={"Total Gallons Schedule"=[], "PRAT/RLT Sequence"=[], "Current Sequence Index"=0}, "Condition Cluster Output"={"Condition #1"=FALSE, "Condition #2"=FALSE, "Special Last Draw (HU Test)"=FALSE, "RTD Out Temperature <="=0.0, "Condition #3"=FALSE, "Mean Tank Temperature <="=0.0, "Condition #4"=FALSE, "Decrease Outlet Temperature \nBy (RTD Out)"=0.0, "Condition #5"=FALSE, "Condition #6"=FALSE, "Time (Seconds)"=0.0, "Condition #7"=FALSE, "Condition #8"=FALSE, "Draw Until Condition"={"UE"=FALSE, "LE"=FALSE, "COMP"=FALSE, "FANS"=FALSE}, "Condition #9"=FALSE}, "HEWH Specific DAQ"={"HEWH Data"={"HEWH Standard"={"Voltage (Volts)"=0.0, "Current (Amps)"=0.0, "Power (Watts)"=0.0, "WattHours (Wh)"=0.0, "TC Tree (AVG)"=0.0, "Flow Rate (GPM)"=0.0, "Gallons (Gal)"=0.0, "RTD Out (Deg F)"=0.0, "RTD In (Deg F)"=0.0, "RTD Amb (Deg F)"=0.0, "TC Down"=0.0, "UE Event Lead"=0, "LE Event Lead"=0, "TC Tree Array"=[]}, "PRAT"={"Power (Watts) A"=4192.0, "Power (Watts) B"=4192.0, "Power (Watts) C"=4192.0, "Power (Watts) D"=4192.0, "TC1"=0.0, "TC2"=0.0, "TC3"=0.0, "TC4"=0.0, "WattHours (Wh) A"=4192.0, "WattHours (Wh) B"=4192.0, "WattHours (Wh) C"=4192.0, "WattHours (Wh) D"=4192.0, "Ambient"=0.0, "Extra Temp"=0.0}, "Additional Power Data"={"Vthd"=236.2, "Frequency (Hz)"=236.2, "Apparent Power (VA)"=236.2, "Power Factor"=236.2, "Current Crest Factor"=236.2, "Voltage Crest Factor"=236.2, "Integration Time (sec)"=236.2}}, "Intellif Valve % Open"=0.0, "Power State"={"UE"=FALSE, "LE"=FALSE, "COMP"=FALSE, "FANS"=FALSE}, "Power Analyzer"=enum."APLUS", "Intellifaucet Configuration"=enum."DRK375,STATION3,1/2\"HOSE"}, "Test Output Data"={"PreDraw Data Table"=[], "Data Table"=[], "MW100 TC Headers"=[]}, "Calc and Calibration"={"RTD Max Min Array"=[], "Draw Statistics"=[], "Calibration Coefficients DBL"=[], "Min RTD Temp\nDuring Draw"=0.0, "Start Gallons"=0.0, "Starting Temp Decline Temp"=0.0, "Max RTD Temp\nDuring Draw"=0.0, "Draw Start Time"=0.0, "Delay Start Time"=0.0, "Current Purge Start Time"=0.0}, "Current Draw Time"=0.0}  # HEWH Output Information
        w107 = T41 {"Measured IMC"=7.0, "Actual RMC"=7.0, "RMC (Desired)"=100.0, "Bone Dry Wt(lbs)"=7.0, "Tolerance(%)"=5.0}  # Weights
        w108 = T42 {"Current VI Reference"=refnum, "Close Panel on Exit?"=FALSE}  # Core
        w109 = FALSE  # Error Flag
        n44 = Bundle("Core"=w108, "Error Flag"=w109, "Weights"=w107, "HEWH Output Information"=w106, "Test_Type:"="Test_Type:", "Supply Voltage"="Supply Voltage", "Appliance Details"="Appliance Details") -> (w111:T40)  [unwired: 1 in]
        n45 = call <vilib>:"Add State(s) to Queue__jki_lib_state_machine.vi"("State(s) in (\"\")"=w113) -> ("States Out"=w112:string)  [unwired: 14 in]
      }
      frame "Data: Cleanup" {
        # "Cleanup any data and references, here.\n(this is called automatically, by the Macro: Exit)"
        n46 = Unbundle By Name(w114) -> ("Core.Current VI Reference"=w117:refnum<vi>)
        n47 = Close Reference(reference=w117, error in (no error)=w116) -> (error out=w115:errorcluster)
        n48 = call <vilib>:"Add State(s) to Queue__jki_lib_state_machine.vi"("State(s) in (\"\")"=w119) -> ("States Out"=w118:string)  [unwired: 14 in]
      }
      frame "---------- UI ----------" {
        # "Do not put any code in this frame.\n(It is a separator no-op. You can make a copy of this frame to create a new UI frame)"
        n49 = call <vilib>:"Add State(s) to Queue__jki_lib_state_machine.vi"("State(s) in (\"\")"=w123) -> ("States Out"=w122:string)  [unwired: 14 in]
      }
      frame "UI: Initialize" {
        n50 = Format Date/Time String(time format string (%c)="Date_%m_%d_%Y_Time_%H_%M_") -> (date/time string=w126:string)  [unwired: 2 out]
        n51 = call "UTILITY IP and Computer Name.vi"() -> ("IP Address"=w124:string, "Computer Name"=w125:string)  [unwired: 10 in]
        n52 = Bundle By Name(cluster=w129, "Date:"=w126, "Computer:"=w125, "Computer IP Address:"=w124) -> (w128:T40)
        n53 = call <vilib>:"Add State(s) to Queue__jki_lib_state_machine.vi"("State(s) in Front (\"\")"="UI: Front Panel State >> Close", "State(s) in (\"\")"=w133) -> ("States Out"=w132:string)  [unwired: 13 in]
      }
      frame "UI: Cursor Set" {
        # "Argument"
        # "Set and Unset Cursor Busy.\n(Usage: \"UI: Cursor Set >> Busy|Idle\")"
        n54 = case shown="\"Idle\", Default" w134 {
          tunnel: w136 -> [w141 w143]
          tunnel: [w140 w142] -> w135
          frame "Idle", Default {
            n55 = call <vilib>:"Unset Busy.vi"("error in (no error)"=w141) -> ("error out"=w140:errorcluster)  [unwired: 10 in]
          }
          frame "Busy" {
            n56 = call <vilib>:"Set Busy.vi"("error in (no error)"=w143) -> ("error out"=w142:errorcluster)  [unwired: 9 in, 1 out]
          }
        }
        n57 = call <vilib>:"Add State(s) to Queue__jki_lib_state_machine.vi"("State(s) in (\"\")"=w139) -> ("States Out"=w138:string)  [unwired: 14 in]
      }
      frame "Update Station" {
        n58 = local write "Test Station"("Station") -> ()
        n59 = Bundle By Name(cluster=w146, "Test Station:"="Station") -> (w145:T40)
        n60 = call <vilib>:"Add State(s) to Queue__jki_lib_state_machine.vi"("State(s) in (\"\")"=w149) -> ("States Out"=w148:string)  [unwired: 14 in]
      }
      frame "UI: Front Panel State" {
        # "Argument"
        # "Set Front Panel Open or Closed\n(Usage: \"UI: Front Panel State >> Open|Close\")"
        n61 = Unbundle By Name(w152) -> ("Core.Current VI Reference"=w151:refnum<vi>)
        n62 = case shown="\"Close\"" w150 {
          tunnel: w154 -> [w160 w173]
          tunnel: [w162 w174] -> w153
          tunnel: w151 -> [w161 w171]
          frame "Open", Default {
            n63 = property class="VI"(reference=w161, error in=w160) -> (reference out=w158:refnum<vi>, error out=w159:errorcluster, "Front Panel.Open"=w157:bool)
            n64 = case shown="False" w157 {
              tunnel: [w165 w168] -> w162
              tunnel: w159 -> [w164 w168]
              tunnel: w158 -> [w163 _]
              frame False {
                n65 = invoke class="VI" method="FP.Open"(reference=w163, error in=w164, "Activate"=TRUE, "State"=T17."Standard") -> (error out=w165:errorcluster)  [unwired: 1 in, 4 out]
              }
              frame True {
              }
            }
          }
          frame "Close" {
            n66 = property class="VI"(reference=w171, error in=w173) -> (reference out=w170:refnum<vi>, error out=w172:errorcluster, "Front Panel.Open"=w169:bool)
            n67 = case shown="True" w169 {
              tunnel: [w175 w178] -> w174
              tunnel: w172 -> [w175 w177]
              tunnel: w170 -> [_ w176]
              frame False {
              }
              frame True {
                n68 = invoke class="VI" method="FP.Close"(reference=w176, error in=w177) -> (error out=w178:errorcluster)  [unwired: 1 in, 2 out]
              }
            }
          }
        }
        n69 = call <vilib>:"Add State(s) to Queue__jki_lib_state_machine.vi"("State(s) in (\"\")"=w156) -> ("States Out"=w155:string)  [unwired: 14 in]
      }
      frame "---------- Macro ----------" {
        n70 = call <vilib>:"Add State(s) to Queue__jki_lib_state_machine.vi"("State(s) in (\"\")"=w182) -> ("States Out"=w181:string)  [unwired: 14 in]
      }
      frame "Macro: Initialize" {
        w183 = "" ("Dryer Type:")
        n71 = property on="OK" class="Bool"("Key Focus"=FALSE) -> ()  [unwired: 2 in, 2 out]
        n72 = local write "Build:"(w183) -> ()
        n73 = local write "Heating Mode:"(w183) -> ()
        n74 = call <vilib>:"Add State(s) to Queue__jki_lib_state_machine.vi"("State(s) in Front (\"\")"="Data: Initialize\nUpdate Station\nInitialize Core Data\nUI: Initialize", "State(s) in (\"\")"=w189) -> ("States Out"=w188:string)  [unwired: 13 in]
      }
      frame "Macro: Exit" {
        n75 = Unbundle By Name(w196) -> ("Core.Close Panel on Exit?"=w190:bool)
        n76 = Select(t="UI: Front Panel State >> Close", s=w190, f="") -> (s? t:f=w193:string)
        n77 = call <vilib>:"Add State(s) to Queue__jki_lib_state_machine.vi"("State(s) in (\"\")"=w193, "State(s) at Back (\"\")"="Data: Cleanup\nExit") -> ("States Out"=w191:string)  [unwired: 13 in]
        n78 = call <vilib>:"Add State(s) to Queue__jki_lib_state_machine.vi"("State(s) in Front (\"\")"=w191, "State(s) in (\"\")"=w199) -> ("States Out"=w198:string)  [unwired: 13 in]
      }
      frame "---------- New Category ----------" {
        n79 = call <vilib>:"Add State(s) to Queue__jki_lib_state_machine.vi"("State(s) in (\"\")"=w203) -> ("States Out"=w202:string)  [unwired: 14 in]
      }
      frame "Get New Info" {
        n80 = local read "Supply Voltage"() -> (w212:string)
        n81 = Bundle By Name(cluster=w221, "Appliance Details.Appliance Common.TR Number:"="TR Number:", "Appliance Details.Appliance Common.Lab ID:"="Lab ID:", "Test Number:"="Test Name:", "Model:"="Model:", "Appliance Details.Appliance Common.Serial Number:"="Serial Number:", "Ambient Temp SetPoint:"="Ambient Temp SetPoint:", "Appliance Details.Appliance Common.Ambient RH:"="Ambient RH:", "Test Station:"="Test Station", "Supply Voltage"=w212, "Appliance Details.Appliance Common.Frequency:"="Frequency:", "Appliance Details.Appliance Common.Engineer:"="Engineer:", "Appliance Details.Appliance Common.Technician:"="Technician:", "Appliance Details.Appliance Common.Build:"="Build:", "Heating Mode"="Heating Mode:", "Appliance Details.Appliance Common.Comments:"="Comments:") -> (w220:T40)
        n82 = call <vilib>:"Add State(s) to Queue__jki_lib_state_machine.vi"("State(s) in (\"\")"=w219) -> ("States Out"=w223:string)  [unwired: 14 in]
      }
      frame "Check Contents" {
        # "If all of the data fields have information go ahead and generate the filename"
        n83 = Unbundle By Name(w242) -> ("Appliance Details.Appliance Common.TR Number:"=w240:string, "Appliance Details.Appliance Common.Lab ID:"=w239:string, "Test Number:"=w238, "Model:"=w237, "Appliance Details.Appliance Common.Serial Number:"=w236:string, "Ambient Temp SetPoint:"=w235, "Appliance Details.Appliance Common.Ambient RH:"=w234:string, "Test Station:"=w233, "Supply Voltage"=w232:string, "Appliance Details.Appliance Common.Frequency:"=w231:string, "Appliance Details.Appliance Common.Engineer:"=w230:string, "Appliance Details.Appliance Common.Technician:"=w229:string, "Appliance Details.Appliance Common.Build:"=w228:string, "Heating Mode"=w227)
        n84 = Build Array(w240, w239, w238, w237, w236, w235, w234, w233, w232, w231, w230, w229, w228, w227) -> (w226:string[])
        n85 = for {
          tunnel: w226 -> [w248] mode=indexing
          tunnel: [w247] -> w225 mode=indexing
          n86 = String Length(string=w248) -> (length=w249:i32)
          n87 = Greater Than 0?(x=w249) -> (x > 0?=w247:bool)
        }
        n88 = And Array Elements(Boolean array=w225) -> (logical AND=w224:bool)
        n89 = case shown="True" w224 {
          tunnel: ["" "Generate Filename\nGenerate Header Data"] -> w243
          tunnel: w242 -> [w250 w254]
          tunnel: [w250 w254] -> w241
          frame False {
            n90 = One Button Dialog(message="All Test Data Must be Filled In") -> ()  [unwired: 1 in, 1 out]
          }
          frame True {
          }
        }
        n91 = call <vilib>:"Add State(s) to Queue__jki_lib_state_machine.vi"("State(s) in Front (\"\")"=w243, "State(s) in (\"\")"=w246) -> ("States Out"=w245:string)  [unwired: 13 in]
      }
      frame "Generate Filename" {
        # "Generate the filename"
        n92 = Unbundle By Name(w259) -> ("Appliance Details"=w257:T1)  [unwired: 1 out]
        n93 = call "Save File DOE Create Filename Sub.vi"("LV Program"=Save_File_DOE_LabView_Program."HEWH", "Appliance Details"=w257) -> ()  [unwired: 7 in, 3 out]
        n94 = call <vilib>:"Add State(s) to Queue__jki_lib_state_machine.vi"("State(s) in (\"\")"=w261) -> ("States Out"=w260:string)  [unwired: 14 in]
        n95 = Bundle By Name(cluster=w259) -> (w258:T40)  [unwired: 2 in]
      }
      frame "Generate Header Data" {
        # "Check to make sure everything is calibrated\nIf its not, display a message to the user.\n\nAdd a calibration file path from a config file"
        # "This puts all of the entered data into\nan array to be placed on the final output sheet"
        n96 = Unbundle By Name(w268) -> ("HEWH Output Information"=w266:T30, "Test_Type:"=w270:string, "Supply Voltage"=w269:string)
        n97 = call "HEWH Create Header File.vi"("Supply Voltage:"=w269, "Test_Type:"=w270, "HEWH Output Information"=w266) -> ("File Initialization Array"=w265:string[][])  [unwired: 8 in]
        n98 = call "Calibration.vi"("error in (no error)"=w272, "Calibration File Path"=path "C:/Work/Calibration.csv" ("file path (dialog if empty)")) -> ("error out"=w271:errorcluster, "Calibration Data"=w263:string[][])  [unwired: 8 in]
        "OutputData" <- w263
        n99 = Bundle By Name(cluster=w268, "File Initialization Array"=w265, "Calibration Array"=w263) -> (w267:T40)
        n100 = call <vilib>:"Add State(s) to Queue__jki_lib_state_machine.vi"("State(s) in Front (\"\")"="Macro: Exit" ("State(s) in Front (\"\")"), "State(s) in (\"\")"=w274) -> ("States Out"=w273:string)  [unwired: 13 in]
      }
    }
  }
  "error out" <- w6
  n101 = Unbundle By Name(w1) -> ("HEWH Output Information"=→"FileInit Cluster":T30)
